vi "Photonics Measurements Launcher.vi"() -> ()   [LabVIEW 2019]
uses:
  Subsystems/Measurement/Typedefs/Measurement.Type--Enum.ctl
  Subsystems/Measurement/Typedefs/Configuration.SMU--Cluster.ctl
  Subsystems/SMU/Typedefs/Configuration--Cluster.ctl
  Subsystems/Measurement/Typedefs/Configuration.LIA--Cluster.ctl
  Subsystems/LIA/Typedefs/Configuration--Cluster.ctl
  Subsystems/Measurement/Typedefs/Configuration.OPM--Cluster.ctl
  Subsystems/OPM/Typedefs/Configuration--Cluster.ctl
  Subsystems/Measurement/Typedefs/Configuration.OPA--Cluster.ctl
  Subsystems/OPA/Typedefs/Configuration--Cluster.ctl
  Subsystems/Measurement/Typedefs/Configuration.XYStage--Cluster.ctl
  Subsystems/XYStage/Typedefs/Configuration--Cluster.ctl
  Subsystems/Measurement/Typedefs/Configuration.MC--Cluster.ctl
  Subsystems/MC/Typedefs/Configuration--Cluster.ctl
  Subsystems/Measurement.IVCurve/Typedefs/Configuration.Measurement--Cluster.ctl
  Subsystems/Measurement.WavelengthSweeping/Typedefs/Configuration.Measurement--Cluster.ctl
  Subsystems/Measurement.PhotocurrentMapping/Typedefs/Configuration.Measurement--Cluster.ctl
  Subsystems/Measurement.PhotocurrentMapping/Typedefs/Configuration.Axis--Cluster.ctl
  Subsystems/Measurement.Free/Measurement.Free.lvclass
  E:/UPWORK/Laser Tool/Laser/project/Subsystems/Measurement/Measurement.lvclass
  Subsystems/Measurement.Free.UI/Measurement.Free.UI.lvclass
  E:/UPWORK/Laser Tool/Laser/project/Subsystems/Measurement.UI/Measurement.UI.lvclass
  Subsystems/Measurement.IVCurve/Measurement.IVCurve.lvclass
  Subsystems/Measurement.IVCurve.UI/Measurement.IVCurve.UI.lvclass
  Subsystems/Measurement.WavelengthSweeping/Measurement.WavelengthSweeping.lvclass
  Subsystems/Measurement.WavelengthSweeping.UI/Measurement.WavelengthSweeping.UI.lvclass
  Subsystems/Measurement.PhotocurrentMapping/Measurement.PhotocurrentMapping.lvclass
  Subsystems/Measurement.PhotocurrentMapping.UI/Measurement.PhotocurrentMapping.UI.lvclass
  Subsystems/Measurement.Free/Typedefs/Configuration--Cluster.ctl
  Subsystems/Measurement.Free/Typedefs/Configuration.Hardware--Cluster.ctl
  Subsystems/Measurement.IVCurve/Typedefs/Configuration--Cluster.ctl
  Subsystems/Measurement.IVCurve/Typedefs/Configuration.Hardware--Cluster.ctl
  Subsystems/Measurement.WavelengthSweeping/Typedefs/Configuration--Cluster.ctl
  Subsystems/Measurement.WavelengthSweeping/Typedefs/Configuration.Hardware--Cluster.ctl
  Subsystems/Measurement.PhotocurrentMapping/Typedefs/Configuration--Cluster.ctl
  Subsystems/Measurement.PhotocurrentMapping/Typedefs/Configuration.Hardware--Cluster.ctl
  Subsystems/Measurement/Measurement.lvclass
  Subsystems/OPA.OrpheusHP/OPA.OrpheusHP.lvclass
  Subsystems/OPM.ThorlabsPM400/OPM.ThorlabsPM400.lvclass
  Subsystems/SMU/SMU.lvclass
  Subsystems/OPA/OPA.lvclass
  Subsystems/OPM/OPM.lvclass
  Subsystems/LIA/LIA.lvclass
  Subsystems/XYStage.KIM101/XYStage.KIM101.lvclass
  Subsystems/XYStage/XYStage.lvclass
  Subsystems/MC/MC.lvclass
panel:
  in  "OK":bool
  out "Measurements Tree":string(tree) caption="Chart A"
  in  "Add":bool
  in  "Remove":bool
  in  "Stop":bool
  in  "Start":bool
  in  "Measurement Parameters":T1(tab)
  in  "SMU step voltage, V":dbl=0.01 min=0.0 step=0.01 format="%.4f"
  in  "SMU stop voltage, V":dbl=2.0 min=0.0 step=0.01 format="%.4f"
  in  "SMU start voltage, V":dbl=1.0 min=0.0 step=0.01 format="%.4f"
  in  "I/V Curve Accumulation":u16=5 caption="Accumulation" step=1
  in  "Delay time, ms":u16=500 step=100
  in  "Monochromator\nwavelength offset, nm":dbl=50.0 step=20.0 format="%#_6f"
  in  "Delay time, ms":u16=500 step=100
  in  "W-Sweep Accumulation":u16=5 caption="Accumulation" step=1
  in  "Integration time, s":dbl=5.0 step=0.1
  in  "OPA number of points":u16 step=1
  in  "Scan resolution, nm":dbl=20.0 step=10.0 format="%#_6f"
  in  "Stop wavelength, nm":dbl=1000.0 step=20.0 format="%#_6f"
  in  "Start wavelength, nm":dbl=600.0 step=20.0 format="%#_6f"
  in  "SMU voltage, V":dbl=1.0 step=0.01 format="%#_6f"
  in  "P-Map Accumulation":u16=5 caption="Accumulation" step=1
  in  "Real world units":string="um"
  in  "Counts per unit":u32=1 step=100
  in  "Y Axis Step, units":dbl=250.0 step=100.0 format="%#_6f"
  in  "Y Axis Stop, units":dbl=10000.0 step=100.0 format="%#_6f"
  in  "Y Axis Start, units":dbl=-10000.0 step=100.0 format="%#_6f"
  in  "X Axis Step, units":dbl=250.0 step=100.0 format="%#_6f"
  in  "X Axis Stop, units":dbl=10000.0 step=100.0 format="%#_6f"
  in  "X Axis Start, units":dbl=-10000.0 step=100.0 format="%#_6f"
  in  "Sync":bool
  in  "Save":bool
  in  "Hardware Parameters":enum32{"Free"}(tab)
  in  "XYStage Enable":bool caption="XYStage"
  in  "Y Axis":string(combo)="Channel 2"
  in  "X Axis":string(combo)="Channel 1"
  in  "XYStage Refresh List":bool
  in  "XYStage Serial Number":string(combo) caption="Serial Number"
  in  "MC Enable":bool caption="MC"
  in  "MC Resource Name":refnum<visa-resource-name>="COM3" caption="Resource Name"
  in  "OPA Enable":bool caption="OPA"
  in  "OPA Refresh List":bool
  in  "OPA Serial Number":string(combo) caption="Serial Number"
  in  "OPM Enable":bool caption="OPM"
  in  "OPM Refresh List":bool
  in  "OPM Simulated":bool
  in  "OPM Resource Name":string(combo) caption="Resource Name"
  in  "LIA Enable":bool caption="LIA"
  in  "LIA Simulated":bool
  in  "LIA Resource Name":refnum<visa-resource-name>="GPIB0::8::INSTR" caption="Resource Name"
  in  "SMU Enable":bool caption="SMU"
  in  "SMU Channel":string(combo)="A" caption="Channel"
  in  "SMU Simulated":bool
  in  "SMU Resource Name":refnum<visa-resource-name>="GPIB0::26::INSTR" caption="Resource Name"
  in  "Close":bool
  out "Status":string
  out "Progress":u8(slide) scale=0.0..100.0
  # "XY Stage Controller"
  # "Monochromator"
  # "Optical Parametric Amplifier"
  # "Optical Power Monitor"
  # "Lock-In Amplifier"
  # "SMU"
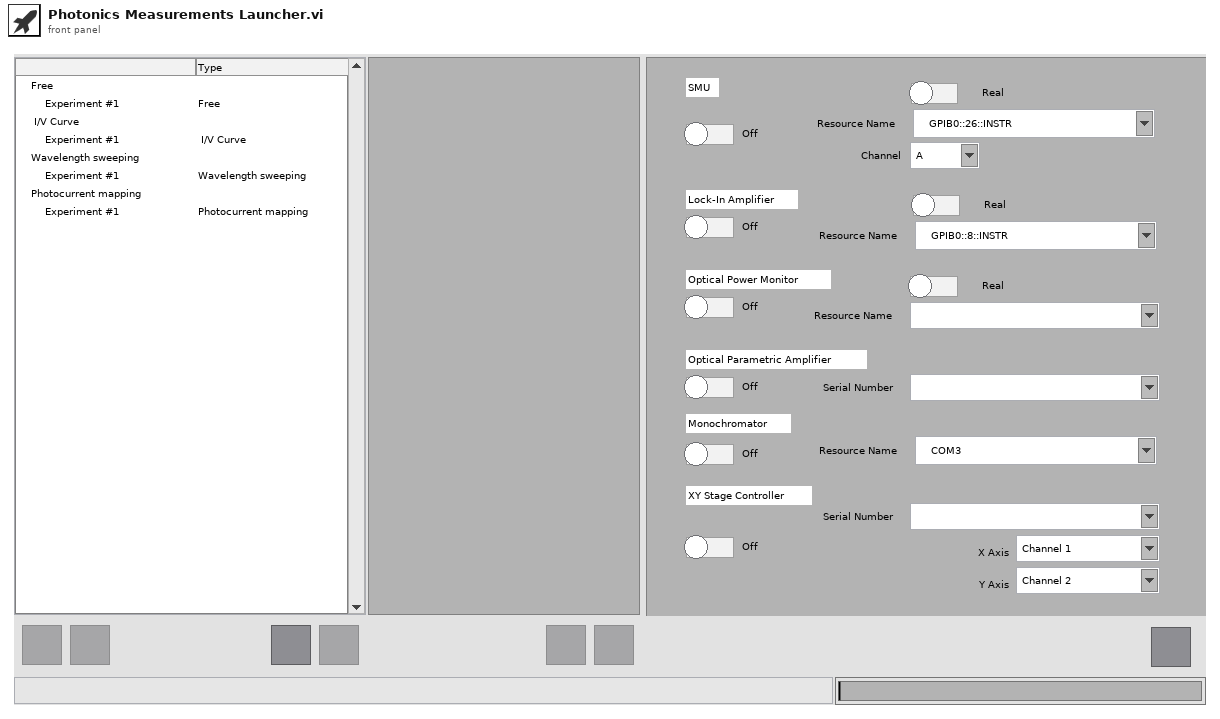
[diagram p1: front panel]
types:
  T1 = enum32{"Free", "I-V Curve", "Wavelength Sweeping", "Photocurrent mapping"}
  T2 = enum8{"Enabled", "Disabled", "Disabled and Grayed Out"}
  T3 = enum32{"Invalid", "Standard", "Closed", "Hidden", "Minimized", "Maximized"}
  T4 = enum32{"invalid app kind", "Development System", "Run Time System", "Student Edition", "Embedded LabVIEW", "Evaluation", "Custom"}
  T5 = typedef "Measurement.lvclass/Measurement.Type--Enum.ctl" = enum16{"Free", "I/V Curve", "Wavelength sweeping", "Photocurrent mapping"}
  T6 = typedef "LVPoint32TypeDef.ctl" = cluster{"Horizontal":i32, "Vertical":i32}
  T7 = typedef "Measurement.lvclass/Configuration.SMU--Cluster.ctl" = cluster{"Enable":bool, "SMU Model":string, "Configuration":T8}
  T8 = typedef "SMU.lvclass/Configuration--Cluster.ctl" = cluster{"VISA Resource":string, "Channel":string}
  T9 = typedef "Measurement.lvclass/Configuration.LIA--Cluster.ctl" = cluster{"Enable":bool, "LIA Model":string, "Configuration":T10}
  T10 = typedef "LIA.lvclass/Configuration--Cluster.ctl" = cluster{"VISA Resource":string}
  T11 = typedef "Measurement.lvclass/Configuration.OPM--Cluster.ctl" = cluster{"Enable":bool, "OPM Model":string, "Configuration":T12}
  T12 = typedef "OPM.lvclass/Configuration--Cluster.ctl" = cluster{"VISA Resource":string}
  T13 = typedef "Measurement.lvclass/Configuration.OPA--Cluster.ctl" = cluster{"Enable":bool, "OPA Model":string, "Configuration":T14}
  T14 = typedef "OPA.lvclass/Configuration--Cluster.ctl" = cluster{"Serial Number":string}
  T15 = typedef "Measurement.lvclass/Configuration.XYStage--Cluster.ctl" = cluster{"Enable":bool, "XYStage Model":string, "Configuration":T16}
  T16 = typedef "XYStage.lvclass/Configuration--Cluster.ctl" = cluster{"Serial Number":string, "X Axis":string, "Y Axis":string, "Real-World Units":string, "Counts per Unit":u32}
  T17 = typedef "Measurement.lvclass/Configuration.MC--Cluster.ctl" = cluster{"Enable":bool, "MC Model":string, "Configuration":T18}
  T18 = typedef "MC.lvclass/Configuration--Cluster.ctl" = cluster{"VISA Resource":string}
  T19 = typedef "Measurement.IVCurve.lvclass/Configuration.Measurement--Cluster.ctl" = cluster{"SMU Voltage Start, V":dbl, "SMU Voltage Stop, V":dbl, "SMU Voltage Step, V":dbl, "Delay time, ms":u16, "Accumulation":u16}
  T20 = typedef "Measurement.WavelengthSweeping.lvclass/Configuration.Measurement--Cluster.ctl" = cluster{"SMU Voltage, V":dbl, "Start wavelength, nm":dbl, "Stop wavelength, nm":dbl, "Scan resolution, nm":dbl, "Number or points":u16, "Integration time, sec":dbl, "Delay time, ms":u16, "Accumulation":u16, "Wavelength offset, nm":dbl}
  T21 = typedef "Measurement.PhotocurrentMapping.lvclass/Configuration.Measurement--Cluster.ctl" = cluster{"X":T22, "Y":T22, "Accumulation":u16}
  T22 = typedef "Measurement.PhotocurrentMapping.lvclass/Configuration.Axis--Cluster.ctl" = cluster{"Start, units":dbl, "Stop, units":dbl, "Step, units":dbl}
  T23 = cluster{"Core":cluster{"Current VI Reference":refnum<vi>, "Close Panel on Exit?":bool}, "Measurements Tree":refnum<vi>, "Measurement.Type":T5, "Configuration (variant)":variant, "Configuration":cluster{"Hardware":cluster{"SMU":T7, "LIA":T9, "OPM":T11, "OPA":T13, "XYStage":T15, "MC":T17}, "Measurement":cluster{"I/V Curve":T19, "W-Sweep":T20, "P-Map":T21}}}
  T24 = cluster{"Hardware":cluster{"SMU":T7, "LIA":T9, "OPM":T11, "OPA":T13, "XYStage":T15, "MC":T17}, "Measurement":cluster{"I/V Curve":T19, "W-Sweep":T20, "P-Map":T21}}
  T25 = cluster{"Current VI Reference":refnum<vi>, "Close Panel on Exit?":bool}
  T26 = typedef "Measurement.Free.lvclass/Configuration--Cluster.ctl" = cluster{"Measurement.Type":T5, "Hardware":T27}
  T27 = typedef "Measurement.Free.lvclass/Configuration.Hardware--Cluster.ctl" = cluster{"SMU":T7, "LIA":T9, "OPM":T11, "OPA":T13, "MC":T17}
  T28 = typedef "Measurement.IVCurve.lvclass/Configuration--Cluster.ctl" = cluster{"Measurement.Type":T5, "Hardware":T29, "Measurement":T19}
  T29 = typedef "Measurement.IVCurve.lvclass/Configuration.Hardware--Cluster.ctl" = cluster{"SMU":T7}
  T30 = typedef "Measurement.WavelengthSweeping.lvclass/Configuration--Cluster.ctl" = cluster{"Measurement.Type":T5, "Hardware":T31, "Measurement":T20}
  T31 = typedef "Measurement.WavelengthSweeping.lvclass/Configuration.Hardware--Cluster.ctl" = cluster{"SMU":T7, "LIA":T9, "OPM":T11, "OPA":T13, "MC":T17}
  T32 = typedef "Measurement.PhotocurrentMapping.lvclass/Configuration--Cluster.ctl" = cluster{"Measurement.Type":T5, "Hardware":T33, "Measurement":T21}
  T33 = typedef "Measurement.PhotocurrentMapping.lvclass/Configuration.Hardware--Cluster.ctl" = cluster{"SMU":T7, "LIA":T9, "XYStage":T15}
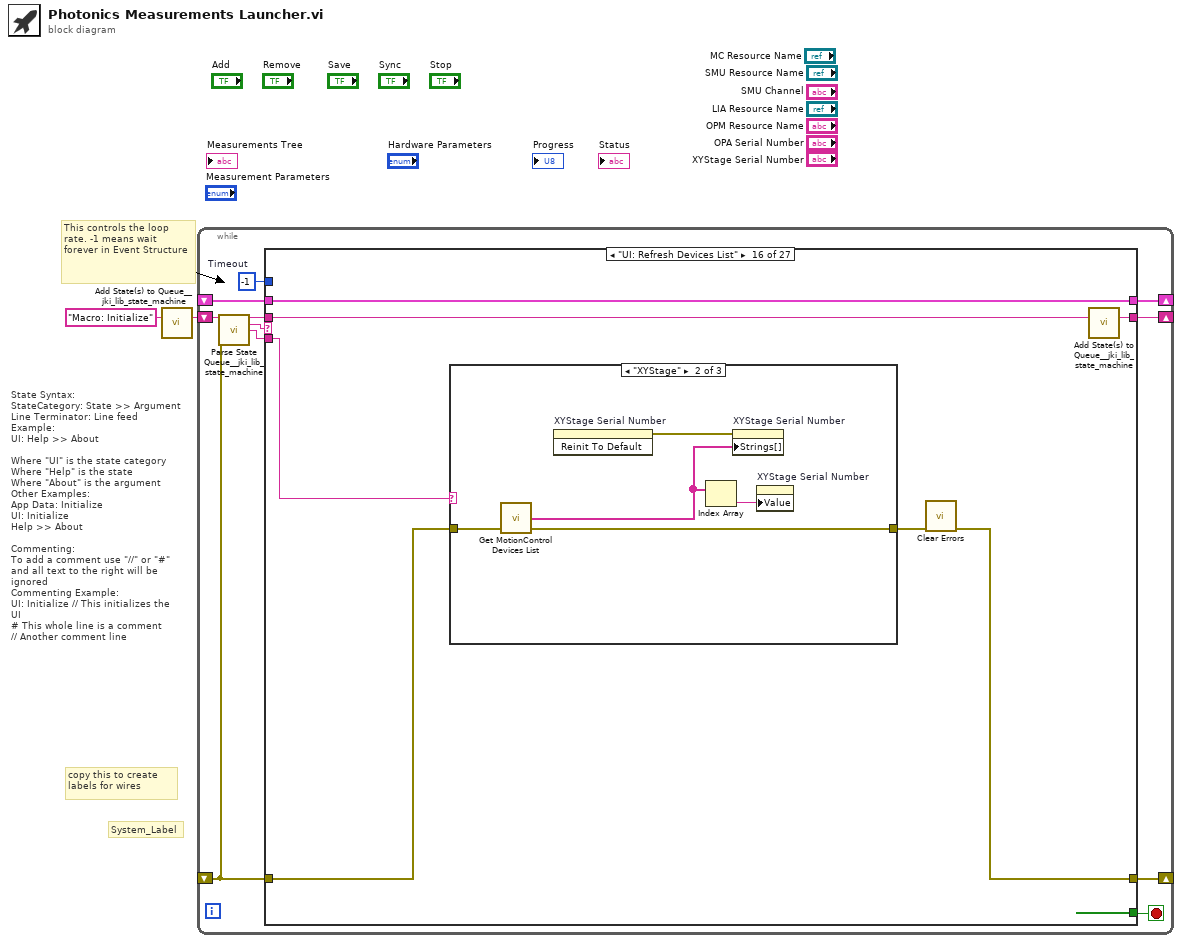
[diagram p0: block diagram]
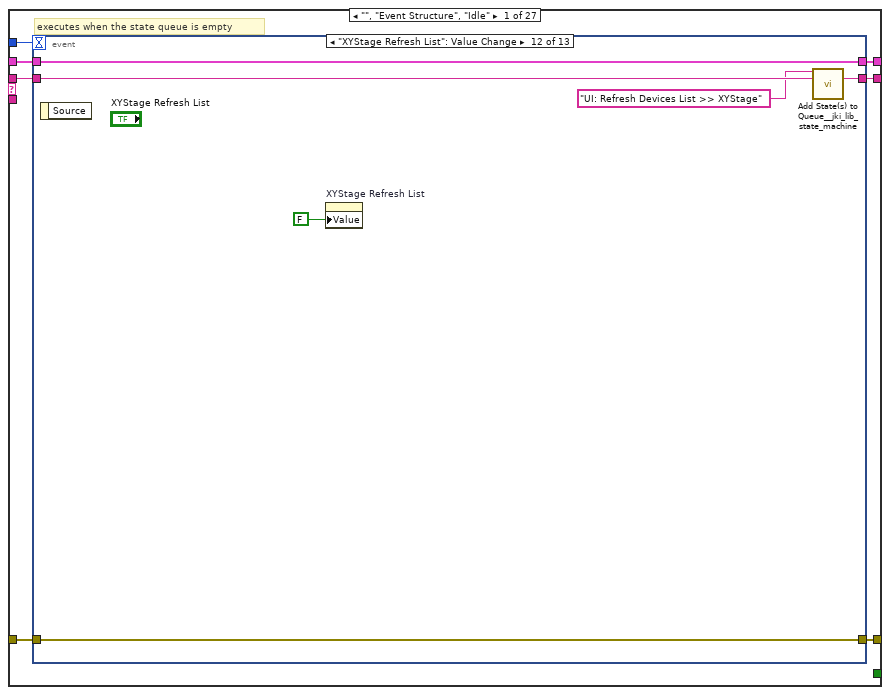
[diagram p2: hidden frame]
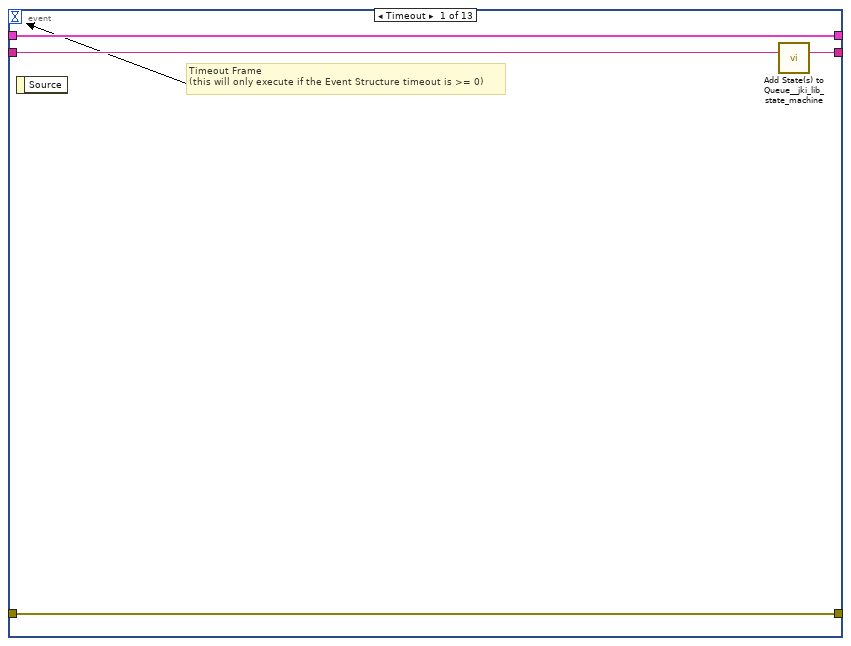
[diagram p3: hidden frame]
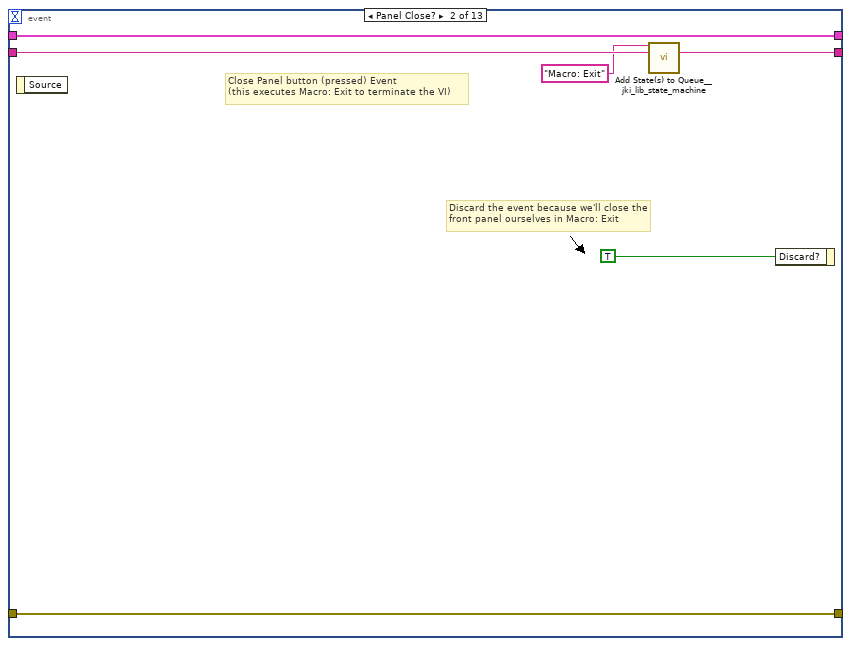
[diagram p4: hidden frame]
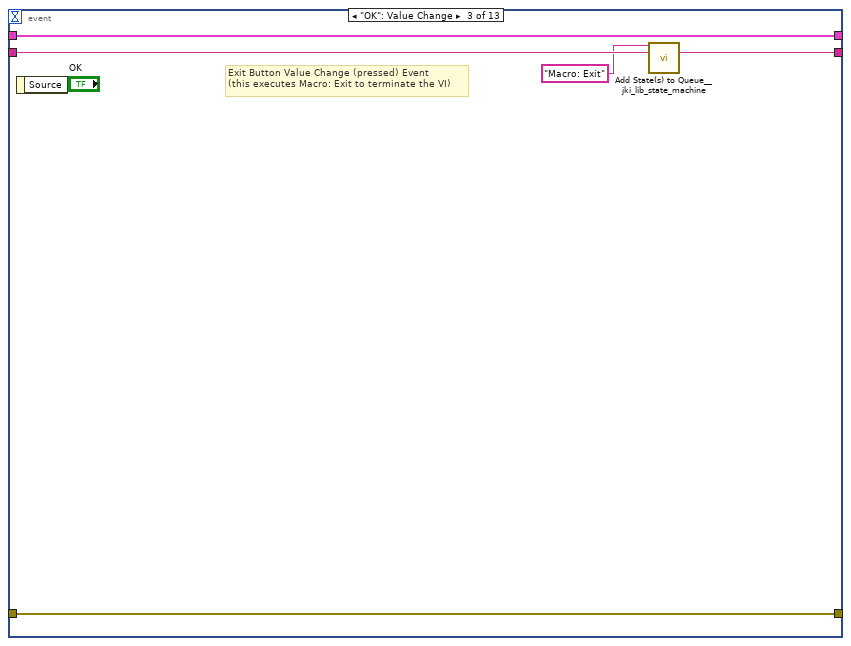
[diagram p5: hidden frame]
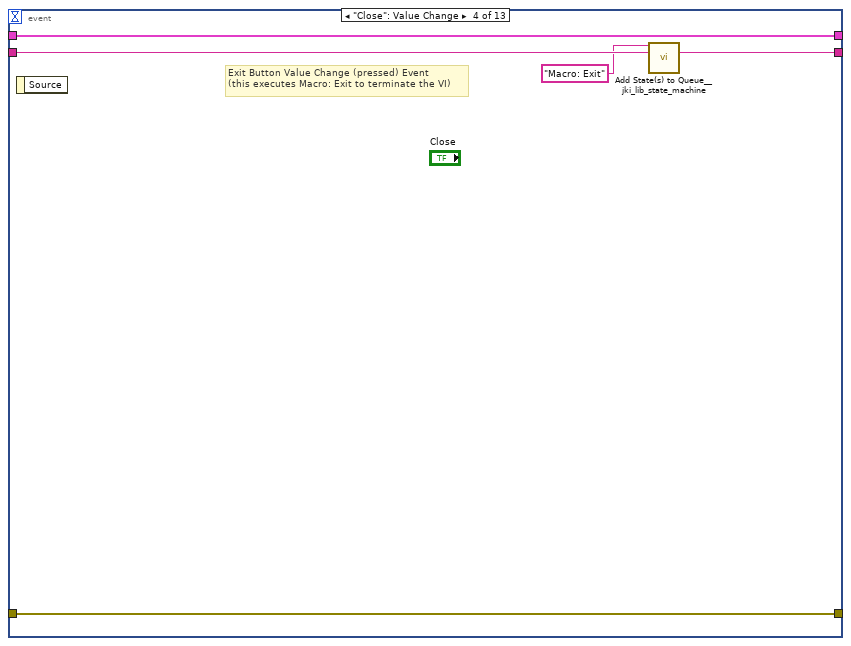
[diagram p6: hidden frame]
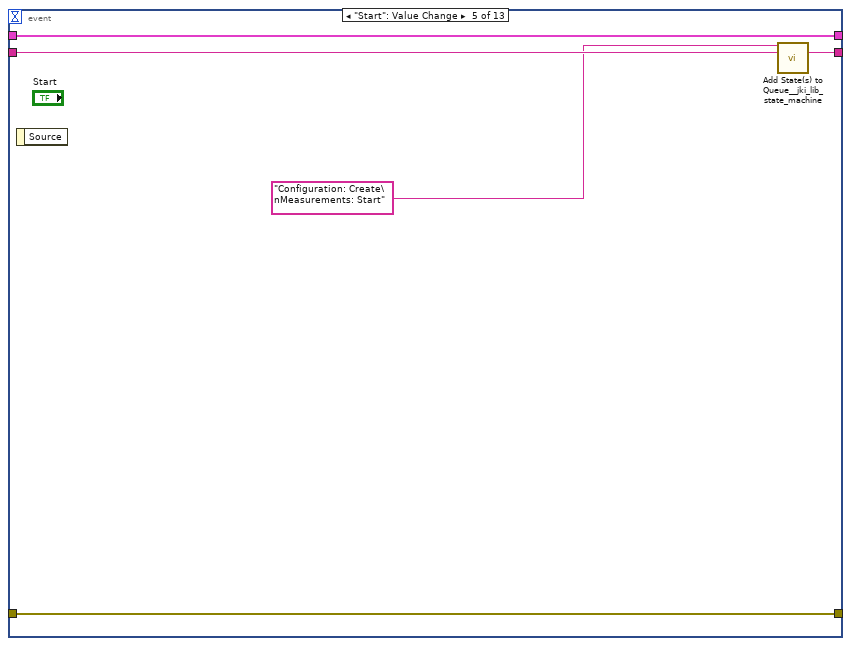
[diagram p7: hidden frame]
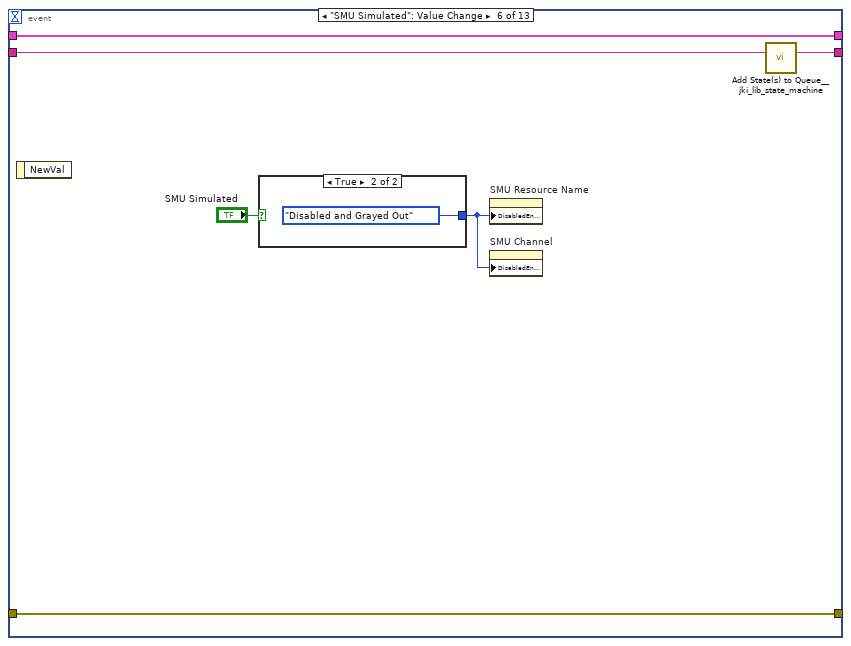
[diagram p8: hidden frame]
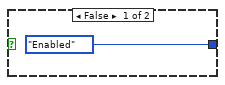
[diagram p9: hidden frame]
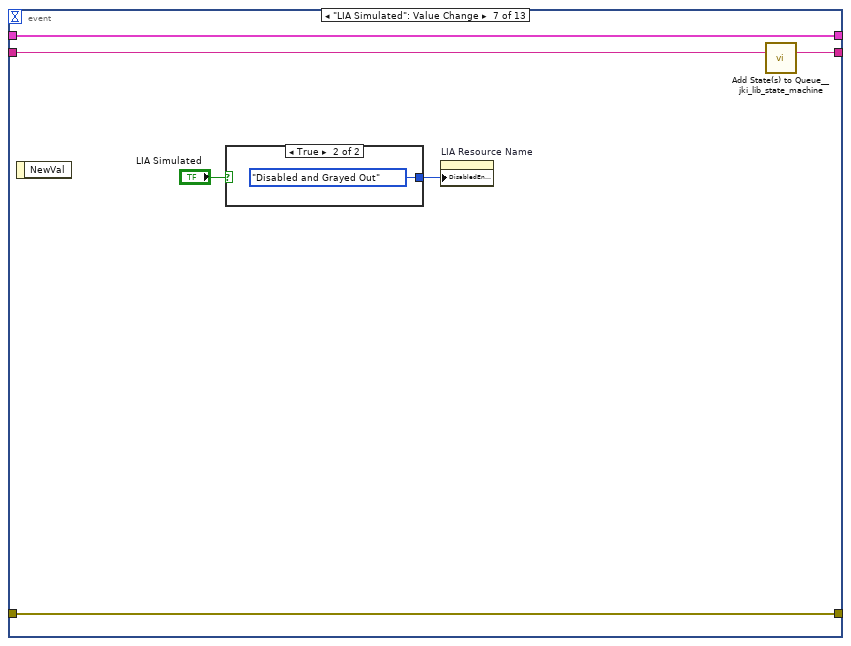
[diagram p10: hidden frame]
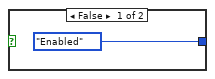
[diagram p11: hidden frame]
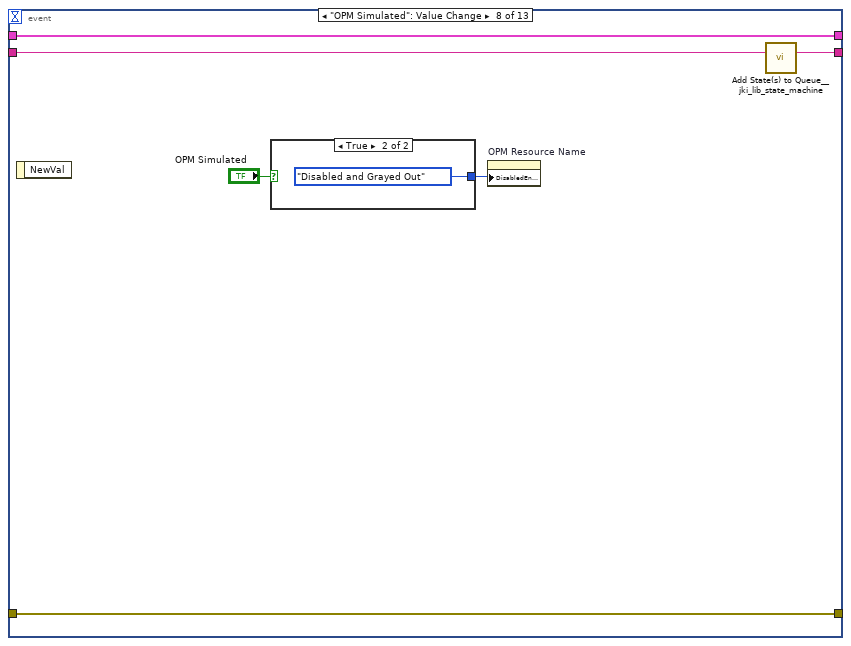
[diagram p12: hidden frame]
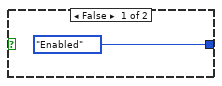
[diagram p13: hidden frame]
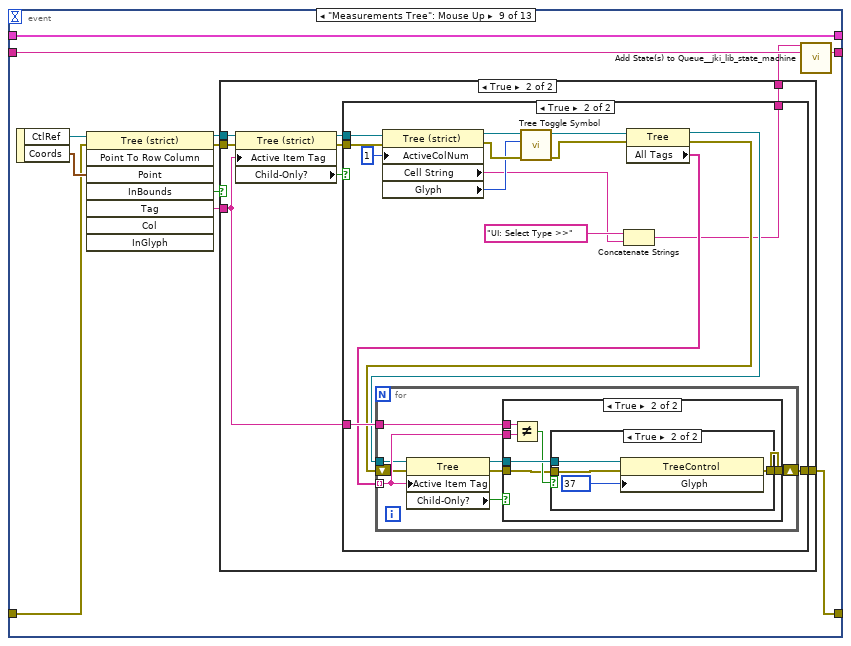
[diagram p14: hidden frame]
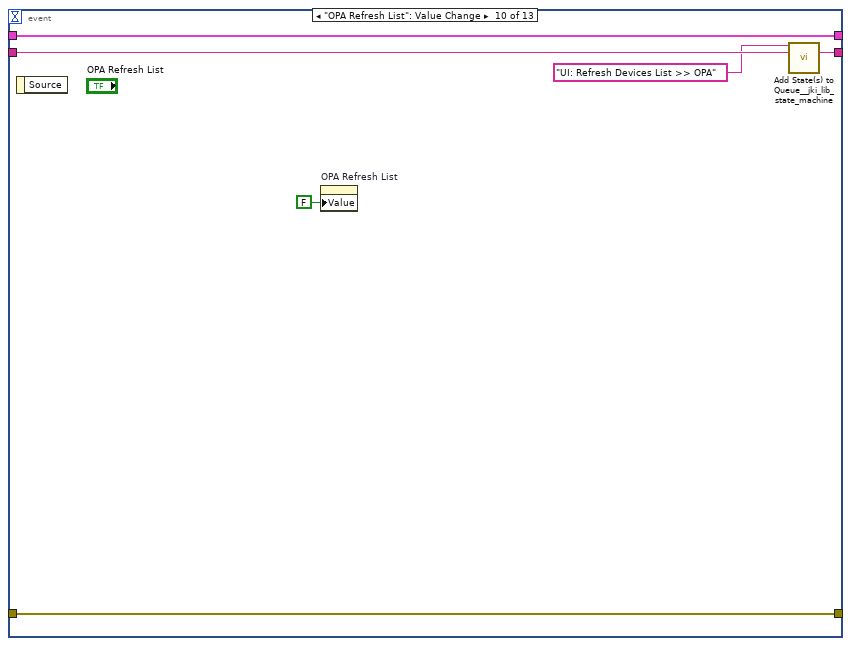
[diagram p19: hidden frame]
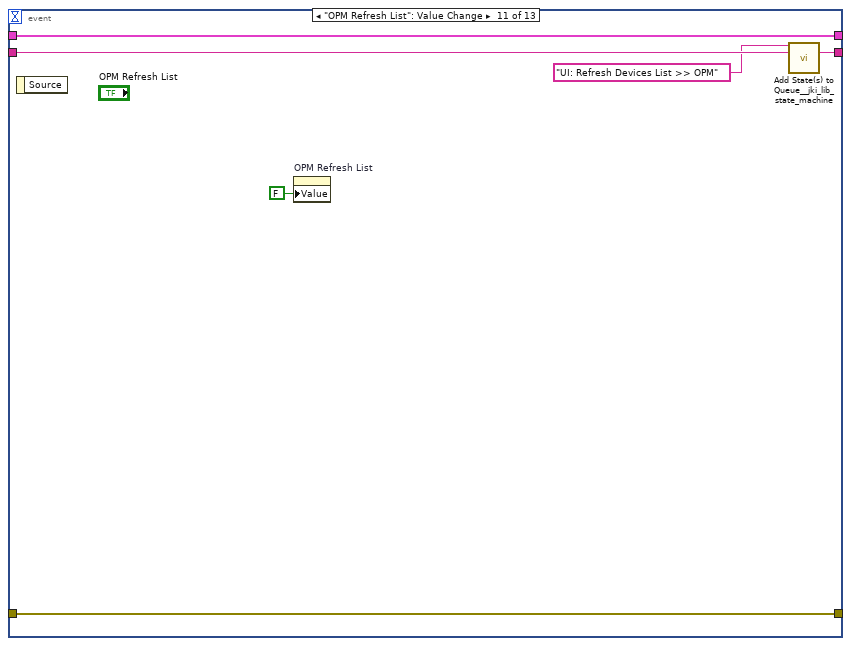
[diagram p20: hidden frame]
diagram:
  # "State Syntax:\nStateCategory: State >> Argument\nLine Terminator: Line feed\nExample:\nUI: Help >> About\n\nWhere \"UI\" is the state category\nWhere \"Help\" is the state\nWhere \"About\" is the argument\nOther Examples:\nApp Data: Initialize\nUI: Initialize\nHelp >> About\n\nCommenting:\nTo add a comment use \"//\" or \"#\" and all text to the right will be ignored\nCommenting Example:\nUI: Initialize // This initializes the UI\n# This whole line is a comment\n// Another comment line"
  # "copy this to create labels for wires"
  # "This controls the loop rate. -1 means wait forever in Event Structure"
  # "System_Label"
  n1 = call <vilib>:"Add State(s) to Queue__jki_lib_state_machine.vi"("State(s) in (\"\")"="Macro: Initialize") -> ("States Out"=w2:string)  [unwired: 14 in]
  n2 = while {
    shift-right: [w6] -> _
    shift-left: _ -> [w5]
    shift-right: [w9] -> _
    shift-left: _ -> [w3]
    shift-right: [w8] -> _
    shift-left: w2 -> [w10]
    stop <- w7 stop-if-true
    w4 = -1  # Timeout
    n3 = call <vilib>:"Parse State Queue__jki_lib_state_machine.vi"("State Queue"=w10, "Error In (no error)"=w3) -> ("Remaining States"=w12:string, "Current State"=w13:string, "Arguments"=w11:string)  [unwired: 11 in]
    n4 = case shown="\"UI: Refresh Devices List\"" w13 {
      selector: w13 -> [_ _ w158 _ _ _ _ _ _ _ _ _ _ _ _ _ _ _ _ _ _ _ _ _ _ _ _]
      tunnel: w12 -> [w20 w157 w162 w181 w187 w192 w196 w205 w211 w215 w220 w226 w231 w282 w305 w316 w338 w429 w481 w486 w496 w500 w509 w521 w527 w537 w637]
      tunnel: w11 -> [_ _ _ _ _ _ _ _ _ _ _ _ w227 _ w300 w313 w332 w432 _ _ _ _ _ _ _ w534 w634]
      tunnel: w5 -> [w18 w154 w160 w174 w184 w190 w193 _ w206 w212 w218 w223 w228 w279 w303 w314 w334 w431 w478 w483 w493 w497 w507 w518 w524 w533 w633]
      tunnel: [w17 w155 w164 w178 errorcluster {"status"=FALSE, "code"=0, "source"=""} ("error out") w189 w194 w202 w207 w213 w217 w224 w229 w263 w301 w310 w335 w428 w479 w484 w494 w498 w502 w519 w525 w535 w635] -> w9
      tunnel: w3 -> [w16 w155 w163 w178 w183 w189 w194 w202 w208 w213 w217 w224 w229 w268 w302 w312 w336 w428 w479 w484 w494 w498 w503 w519 w525 w535 w635]
      tunnel: [w19 w156 w161 w180 w186 w191 w195 w204 w210 w214 w219 w225 w230 w281 w304 w315 w337 w433 w480 w485 w495 w499 w508 w520 w526 w536 w636] -> w8
      tunnel: [_ _ _ _ _ TRUE _ _ _ _ _ _ _ _ _ _ _ _ _ _ _ _ _ _ _ _ _] -> w7
      tunnel: [w15 w154 w160 w179 w184 w190 w193 w203 w206 w212 w218 w223 w228 w279 w303 w314 w334 w430 w478 w483 w493 w497 w507 w518 w524 w532 w632] -> w6
      tunnel: w4 -> [w14 _ _ _ _ _ _ _ _ _ _ _ _ _ _ _ _ _ _ _ _ _ _ _ _ _ _]
      frame "", "Event Structure", "Idle" {
        # "executes when the state queue is empty"
        n5 = event shown="[11] \"XYStage Refresh List\": Value Change" {
          selector: _ -> [_ _ _ _ _ _ _ _ _ _ _ _ _]
          dyn-events: _ -> [_ _ _ _ _ _ _ _ _ _ _ _ _]
          timeout: w14 -> [_ _ _ _ _ _ _ _ _ _ _ _ _]
          tunnel: w20 -> [w24 w30 w35 w40 w43 w47 w57 w65 w79 w133 w139 w145 w150]
          tunnel: [w23 w29 w34 w39 w44 w48 w58 w66 w80 w132 w138 w144 w151] -> w19
          tunnel: w18 -> [w21 w27 w32 w37 w45 w49 w59 w67 w81 w130 w136 w142 w152]
          tunnel: [w22 w28 w33 w38 w42 w46 w56 w64 w72 w131 w137 w143 w153] -> w17
          tunnel: w16 -> [w22 w28 w33 w38 w42 w46 w56 w64 w71 w131 w137 w143 w153]
          tunnel: [w21 w27 w32 w37 w45 w49 w59 w67 w81 w130 w136 w142 w152] -> w15
          event Timeout {
            # "Timeout Frame\n(this will only execute if the Event Structure timeout is >= 0)"
            n6 = event-data() -> ()  [unwired: 1 in, 1 out]
            n7 = call <vilib>:"Add State(s) to Queue__jki_lib_state_machine.vi"("State(s) in (\"\")"=w24) -> ("States Out"=w23:string)  [unwired: 14 in]
          }
          event Panel Close? {
            # "Discard the event because we'll close the front panel ourselves in Macro: Exit"
            # "Close Panel button (pressed) Event\n(this executes Macro: Exit to terminate the VI)"
            n8 = event-data() -> ()  [unwired: 1 in, 1 out]
            n9 = call <vilib>:"Add State(s) to Queue__jki_lib_state_machine.vi"("State(s) in Front (\"\")"="Macro: Exit", "State(s) in (\"\")"=w30) -> ("States Out"=w29:string)  [unwired: 13 in]
            n10 = event-data("Discard?"=TRUE) -> ()  [unwired: 1 in, 1 out]
          }
          event "OK": Value Change {
            # "Exit Button Value Change (pressed) Event\n(this executes Macro: Exit to terminate the VI)"
            n11 = event-data() -> ()  [unwired: 1 in, 1 out]
            n12 = call <vilib>:"Add State(s) to Queue__jki_lib_state_machine.vi"("State(s) in Front (\"\")"="Macro: Exit", "State(s) in (\"\")"=w35) -> ("States Out"=w34:string)  [unwired: 13 in]
          }
          event "Close": Value Change {
            # "Exit Button Value Change (pressed) Event\n(this executes Macro: Exit to terminate the VI)"
            n13 = event-data() -> ()  [unwired: 1 in, 1 out]
            n14 = call <vilib>:"Add State(s) to Queue__jki_lib_state_machine.vi"("State(s) in Front (\"\")"="Macro: Exit", "State(s) in (\"\")"=w40) -> ("States Out"=w39:string)  [unwired: 13 in]
          }
          event "Start": Value Change {
            n15 = event-data() -> ()  [unwired: 1 in, 1 out]
            n16 = call <vilib>:"Add State(s) to Queue__jki_lib_state_machine.vi"("State(s) in Front (\"\")"="Configuration: Create\nMeasurements: Start" ("State(s) in Front (\"\")"), "State(s) in (\"\")"=w43) -> ("States Out"=w44:string)  [unwired: 13 in]
          }
          event "SMU Simulated": Value Change {
            n17 = event-data() -> ()  [unwired: 1 in, 1 out]
            n18 = case shown="True" "SMU Simulated" {
              tunnel: [T2."Enabled" ("Disabled") T2."Disabled and Grayed Out" ("Disabled")] -> w51
              frame False {
              }
              frame True {
              }
            }
            n19 = property on="SMU Resource Name" class="VISAName"("DisabledEnum"=w51) -> ()  [unwired: 2 in, 2 out]
            n20 = property on="SMU Channel" class="CmbBox"("DisabledEnum"=w51) -> ()  [unwired: 2 in, 2 out]
            n21 = call <vilib>:"Add State(s) to Queue__jki_lib_state_machine.vi"("State(s) in (\"\")"=w47) -> ("States Out"=w48:string)  [unwired: 14 in]
          }
          event "LIA Simulated": Value Change {
            n22 = event-data() -> ()  [unwired: 1 in, 1 out]
            n23 = case shown="True" "LIA Simulated" {
              tunnel: [T2."Enabled" ("Disabled") T2."Disabled and Grayed Out" ("Disabled")] -> w55
              frame False {
              }
              frame True {
              }
            }
            n24 = property on="LIA Resource Name" class="VISAName"("DisabledEnum"=w55) -> ()  [unwired: 2 in, 2 out]
            n25 = call <vilib>:"Add State(s) to Queue__jki_lib_state_machine.vi"("State(s) in (\"\")"=w57) -> ("States Out"=w58:string)  [unwired: 14 in]
          }
          event "OPM Simulated": Value Change {
            n26 = event-data() -> ()  [unwired: 1 in, 1 out]
            n27 = case shown="True" "OPM Simulated" {
              tunnel: [T2."Enabled" ("Disabled") T2."Disabled and Grayed Out" ("Disabled")] -> w63
              frame False {
              }
              frame True {
              }
            }
            n28 = property on="OPM Resource Name" class="CmbBox"("DisabledEnum"=w63) -> ()  [unwired: 2 in, 2 out]
            n29 = call <vilib>:"Add State(s) to Queue__jki_lib_state_machine.vi"("State(s) in (\"\")"=w65) -> ("States Out"=w66:string)  [unwired: 14 in]
          }
          event "Measurements Tree": Mouse Up {
            n30 = event-data() -> ("CtlRef"=w78:refnum<vi>, "Coords"=w77:T6)  [unwired: 1 in]
            n31 = invoke class="Tree (strict)" method="Point To Row Column"(reference=w78, error in=w71, "Point"=w77) -> (reference out=w75:refnum<vi>, error out=w74:errorcluster, "InBounds"=w76:bool, "Tag"=w73:string)  [unwired: 5 in, 4 out]
            n32 = case shown="True" w76 {
              tunnel: w75 -> [_ w90]
              tunnel: w74 -> [w82 w89]
              tunnel: w73 -> [_ w85]
              tunnel: [w82 w84] -> w72
              tunnel: [_ w83] -> w70
              frame False {
              }
              frame True {
                n33 = property class="Tree (strict)"(reference=w90, error in=w89, "Active Item Tag"=w85) -> (reference out=w87:refnum<vi>, error out=w86:errorcluster, "Child-Only?"=w88:bool)
                n34 = case shown="True" w88 {
                  tunnel: w87 -> [_ w106]
                  tunnel: w86 -> [w91 w107]
                  tunnel: w85 -> [_ w99]
                  tunnel: [w91 w93] -> w84
                  tunnel: [_ w92] -> w83
                  frame False {
                  }
                  frame True {
                    n35 = property class="Tree (strict)"(reference=w106, error in=w107, "ActiveColNum"=1 ("Active Cell:Active Column Number")) -> (reference out=w104:refnum<vi>, error out=w103:errorcluster, "Cell String"=w100:string, "Glyph"=w102:i32)
                    n36 = call "Tree Toggle Symbol.vi"("error in (no error)"=w103, "Symbol in"=w102, "TreeControl in"=w104) -> ("error out"=w97:errorcluster, "TreeControl out"=w98:refnum<vi>)  [unwired: 5 in, 2 out]
                    n37 = Concatenate Strings("UI: Select Type >>", w100) -> (w92:string)
                    n38 = property class="Tree"(reference=w98, error in=w97) -> (reference out=w96:refnum<vi>, error out=w95:errorcluster, "All Tags"=w94:string[])
                    n39 = for {
                      tunnel: w94 -> [w113] mode=indexing
                      tunnel: w99 -> [w114]
                      tunnel: w96 -> [w111]
                      shift-right: [w108] -> w93
                      shift-left: w95 -> [w110]
                      n40 = property class="Tree"(reference=w111, error in=w110, "Active Item Tag"=w113) -> (reference out=w112:refnum<vi>, error out=w109:errorcluster, "Child-Only?"=w115:bool)
                      n41 = case shown="True" w115 {
                        tunnel: w114 -> [_ w122]
                        tunnel: w113 -> [_ w121]
                        tunnel: w112 -> [_ w120]
                        tunnel: w109 -> [w116 w118]
                        tunnel: [w116 w117] -> w108
                        frame False {
                        }
                        frame True {
                          n42 = Not Equal?(x=w122, y=w121) -> (x != y?=w119:bool)
                          n43 = case shown="True" w119 {
                            tunnel: w120 -> [_ w127]
                            tunnel: w118 -> [w123 w125]
                            tunnel: [w123 w124] -> w117
                            frame False {
                            }
                            frame True {
                              n44 = property class="TreeControl"(reference=w127, error in=w125, "Glyph"=37) -> (error out=w124:errorcluster)  [unwired: 1 out]
                            }
                          }
                        }
                      }
                    }
                  }
                }
              }
            }
            n45 = call <vilib>:"Add State(s) to Queue__jki_lib_state_machine.vi"("State(s) in Front (\"\")"=w70, "State(s) in (\"\")"=w79) -> ("States Out"=w80:string)  [unwired: 13 in]
          }
          event "OPA Refresh List": Value Change {
            n46 = event-data() -> ()  [unwired: 1 in, 1 out]
            n47 = property on="OPA Refresh List" class="Bool (strict)"("Value"=FALSE ("OPA Refresh List")) -> ()  [unwired: 2 in, 2 out]
            n48 = call <vilib>:"Add State(s) to Queue__jki_lib_state_machine.vi"("State(s) in Front (\"\")"="UI: Refresh Devices List >> OPA", "State(s) in (\"\")"=w133) -> ("States Out"=w132:string)  [unwired: 13 in]
          }
          event "OPM Refresh List": Value Change {
            n49 = event-data() -> ()  [unwired: 1 in, 1 out]
            n50 = property on="OPM Refresh List" class="Bool (strict)"("Value"=FALSE ("OPM Refresh List")) -> ()  [unwired: 2 in, 2 out]
            n51 = call <vilib>:"Add State(s) to Queue__jki_lib_state_machine.vi"("State(s) in Front (\"\")"="UI: Refresh Devices List >> OPM", "State(s) in (\"\")"=w139) -> ("States Out"=w138:string)  [unwired: 13 in]
          }
          event "XYStage Refresh List": Value Change {
            n52 = event-data() -> ()  [unwired: 1 in, 1 out]
            n53 = property on="XYStage Refresh List" class="Bool (strict)"("Value"=FALSE ("OPM Refresh List")) -> ()  [unwired: 2 in, 2 out]
            n54 = call <vilib>:"Add State(s) to Queue__jki_lib_state_machine.vi"("State(s) in Front (\"\")"="UI: Refresh Devices List >> XYStage", "State(s) in (\"\")"=w145) -> ("States Out"=w144:string)  [unwired: 13 in]
          }
          event "SMU Enable", "LIA Enable", "OPM Enable", "OPA Enable", "MC Enable", "XYStage Enable": Value Change {
            n55 = event-data() -> ("CtlRef"=w146:refnum<vi>)  [unwired: 1 in]
            n56 = property class="Bool (strict)"(reference=w146) -> ("Caption.Text"=w148:string)  [unwired: 1 in, 2 out]
            n57 = Concatenate Strings("UI: Enable/Disable >> ", w148) -> (w147:string)
            n58 = call <vilib>:"Add State(s) to Queue__jki_lib_state_machine.vi"("State(s) in Front (\"\")"=w147, "State(s) in (\"\")"=w150) -> ("States Out"=w151:string)  [unwired: 13 in]
          }
        }
      }
      frame "---------- Core ----------" {
        # "Do not put any code in this frame.\n(it is a separator no-op)"
        n59 = call <vilib>:"Add State(s) to Queue__jki_lib_state_machine.vi"("State(s) in (\"\")"=w157) -> ("States Out"=w156:string)  [unwired: 14 in]
      }
      frame Default {
        w167 = 42 items=["No error", "Argument error", "Memory is full", "Out of zone", "End of file", "File already open", "Generic file I/O error", "File not found", "File permission error", "Disk is full", "Duplicate path", "Too many files open", "System feature not enabled", "Resource file not found", "Cannot add resource", "Resource not found", "Image not found", "Image memory error", "Pen does not exist", "Config type invalid", "Config token not found", "Config parse error", "Config memory error", "Bad external code format", "Bad external code offset", "External code not present", "Null window", "Destroy window error", "Null menu", "Print aborted", "Bad print record", "Print driver error", "Windows error during printing", "Memory error during printing", "Print dialog error", "Generic print error", "Invalid device refnum", "Device not found", "Device parameter error", "Device unit error", "Cannot open device", "Device call aborted", "Generic error", "Cancelled by user", "Object ID too low", "Object ID too high", "Object not in heap", "Unknown heap", "Unknown object (invalid DefProc)", "Unknown object (DefProc not in table)", "Message out of range", "Invalid (null) method", "Unknown message", "Manager call not supported", "Bad address", "Network operation in progress", "Network operation timed out", "Connection is busy", "Network attribute not supported", "Network error", "Address in use", "System out of memory", "Connection aborted", "Connection refused", "Not connected", "Already connected", "Connection closed", "Initialization error (interapplication manager)", "Bad occurrence", "Wait on unbound occurrence handler", "Occurrence queue overflow", "Datalog type conflict", "Unused", "Unrecognized type (interapplication manager)", "Memory corrupt", "Failed to make temporary DLL", "Old CIN version", "Drag socket not found", "Failed to load drop-object", "Failed to register OLE object", "Failed to release OLE object", "Format specifier type mismatch", "Unknown format specifier", "Too few format specifiers", "Too many format specifiers", "Scan failed", "Newer CIN version", "Error converting to variant", "Runtime menu error", "Password tampered", "Variant attribute not found", "Incompatible variant data type", "Event data is not available", "Event Store is not present", "Occurrence is not found", "Event Queue is not created", "Event info is not available", "Refnum passed is NULL", "Error retrieving Class GUID", "Error retrieving CoClass GUID", "Error retrieving TypeLib GUID.", "Bad built application magic bytes.", "Specific driver is different from the specific driver associated with the Logical Name.", "There is no session opened to the class driver.", "Max Error", "MAX - Error with config objects", "MAX - Error loading configuration", "MAX - Group not supported"]
        # "Current State"
        # "Do not delete, rename, or modify this frame.\n(this is used to capture unhandled states and typos)"
        # "Handle mistyped state name (developer tool)"
        n60 = Format Into String(format string="Software Exception: Unhandled State \"%s\"." ("message"), error in=w163, w158) -> (resulting string=w166:string, error out=w165:errorcluster)  [unwired: 1 in]
        n61 = call <vilib>:"Error Cluster From Error Code.vi"("show call chain? (False)"=TRUE, "error in (no error)"=w165, "error message (\"\")"=w166, "error code (0)"=w167) -> ("error out"=w164:errorcluster)  [unwired: 5 in]
        n62 = call <vilib>:"Add State(s) to Queue__jki_lib_state_machine.vi"("State(s) in (\"\")"=w162) -> ("States Out"=w161:string)  [unwired: 14 in]
      }
      frame "Initialize Core Data" {
        # "Do not delete, rename, or modify this frame.\n(this is used to determine panel behavior on exit)"
        # "originally closed?"
        # "exe?"
        # "If panel starts closed or is an EXE, then close it when we exit"
        n63 = property class="VI"() -> ("FP.State"=w171:T3)  [unwired: 2 in, 2 out]
        n64 = property class="App"() -> ("App.Kind"=w177:T4)  [unwired: 2 in, 2 out]
        n65 = control-ref of="Current VI Reference"() -> (w172:refnum<vi>)
        n66 = Equal?(x=w171, y=T3."Closed" ("Front Panel Window:State")) -> (x = y?=w169:bool)
        n67 = Equal?(x=w177, y=T4."Run Time System" ("Application:Kind")) -> (x = y?=w175:bool)
        n68 = Or(x=w169, y=w175) -> (x .or. y?=w173:bool)
        n69 = Bundle By Name(cluster=w174, "Core.Current VI Reference"=w172, "Core.Close Panel on Exit?"=w173) -> (w179:T23)
        n70 = call <vilib>:"Add State(s) to Queue__jki_lib_state_machine.vi"("State(s) in (\"\")"=w181) -> ("States Out"=w180:string)  [unwired: 14 in]
      }
      frame "Error Handler" {
        # "Unhandled Error -- Display it"
        # "Handle any errors here.\nYou can also output any states to clean-up after errors occur"
        # "Clear error"
        n71 = call <vilib>:"General Error Handler.vi"("error in (no error)"=w183) -> ()  [unwired: 10 in, 5 out]
        n72 = call <vilib>:"Add State(s) to Queue__jki_lib_state_machine.vi"("State(s) in Front (\"\")"="/* Post Error States", "State(s) in (\"\")"=w187) -> ("States Out"=w186:string)  [unwired: 13 in]
      }
      frame "Exit" {
        # "Do not put any code in this frame.\n(No errors that occur here will be handled.)"
        n73 = call <vilib>:"Add State(s) to Queue__jki_lib_state_machine.vi"("State(s) in (\"\")"=w192) -> ("States Out"=w191:string)  [unwired: 14 in]
      }
      frame "---------- Data ----------" {
        # "Do not put any code in this frame.\n(It is a separator no-op. You can make a copy of this frame to create a new Data frame)"
        n74 = call <vilib>:"Add State(s) to Queue__jki_lib_state_machine.vi"("State(s) in (\"\")"=w196) -> ("States Out"=w195:string)  [unwired: 14 in]
      }
      frame "Data: Initialize" {
        w197 = T24 {"Hardware"={"SMU"={"Enable"=FALSE, "SMU Model"="", "Configuration"={"VISA Resource"="", "Channel"=""}}, "LIA"={"Enable"=FALSE, "LIA Model"="", "Configuration"={"VISA Resource"=""}}, "OPM"={"Enable"=FALSE, "OPM Model"="", "Configuration"={"VISA Resource"=""}}, "OPA"={"Enable"=FALSE, "OPA Model"="", "Configuration"={"Serial Number"=""}}, "XYStage"={"Enable"=FALSE, "XYStage Model"="", "Configuration"={"Serial Number"="", "X Axis"="", "Y Axis"="", "Real-World Units"="", "Counts per Unit"=1}}, "MC"={"Enable"=FALSE, "MC Model"="", "Configuration"={"VISA Resource"=""}}}, "Measurement"={"I/V Curve"={"SMU Voltage Start, V"=0.0, "SMU Voltage Stop, V"=0.0, "SMU Voltage Step, V"=0.0, "Delay time, ms"=0, "Accumulation"=0}, "W-Sweep"={"SMU Voltage, V"=0.0, "Start wavelength, nm"=0.0, "Stop wavelength, nm"=0.0, "Scan resolution, nm"=0.0, "Number or points"=0, "Integration time, sec"=0.0, "Delay time, ms"=0, "Accumulation"=0, "Wavelength offset, nm"=0.0}, "P-Map"={"X"={"Start, units"=-10000.0, "Stop, units"=10000.0, "Step, units"=250.0}, "Y"={"Start, units"=-10000.0, "Stop, units"=10000.0, "Step, units"=250.0}, "Accumulation"=5}}}  # Configuration
        w198 = variant  # Configuration (variant)
        w199 = Measurement.Type--Enum."Free"  # Measurement.Type
        w201 = T25 {"Current VI Reference"=refnum, "Close Panel on Exit?"=FALSE}  # Core
        # "do not delete - used by framework"
        # "Data names and types of shift register data are defined by this bundle."
        # "Initialize the shift-register data, here.\n(data names are defined by what you wire into the bundle function)"
        n75 = control-ref of="Measurements Tree"() -> (w200:refnum<vi>)
        n76 = Bundle("Core"=w201, "Measurements Tree"=w200, "Measurement.Type"=w199, "Configuration (variant)"=w198, "Configuration"=w197) -> (w203:T23)  [unwired: 1 in]
        n77 = call <vilib>:"Add State(s) to Queue__jki_lib_state_machine.vi"("State(s) in (\"\")"=w205) -> ("States Out"=w204:string)  [unwired: 14 in]
      }
      frame "Data: Cleanup" {
        # "Cleanup any data and references, here.\n(this is called automatically, by the Macro: Exit)"
        n78 = Unbundle By Name(w206) -> ("Core.Current VI Reference"=w209:refnum<vi>)
        n79 = Close Reference(reference=w209, error in (no error)=w208) -> (error out=w207:errorcluster)
        n80 = call <vilib>:"Add State(s) to Queue__jki_lib_state_machine.vi"("State(s) in (\"\")"=w211) -> ("States Out"=w210:string)  [unwired: 14 in]
      }
      frame "---------- UI ----------" {
        # "Do not put any code in this frame.\n(It is a separator no-op. You can make a copy of this frame to create a new UI frame)"
        n81 = call <vilib>:"Add State(s) to Queue__jki_lib_state_machine.vi"("State(s) in (\"\")"=w215) -> ("States Out"=w214:string)  [unwired: 14 in]
      }
      frame "UI: Initialize" {
        # "Initialize the User Interface, here.\n(this is called automatically, by the Macro: Init)"
        n82 = call <vilib>:"Add State(s) to Queue__jki_lib_state_machine.vi"("State(s) in Front (\"\")"="UI: Tree Init\nUI: Initial State\nUI: Refresh Devices List >> OPM\nUI: Refresh Devices List >> OPA\nUI: Refresh Devices List >> XYStage\nUI: Select Type >> Free", "State(s) in (\"\")"=w220) -> ("States Out"=w219:string)  [unwired: 13 in]
      }
      frame "UI: Initial State" {
        w221 = FALSE ("SMU Simulated")
        w222 = TRUE ("SMU Enable")
        n83 = property on="SMU Enable" class="Bool (strict)"("Value"=w222) -> ()  [unwired: 2 in, 2 out]
        n84 = property on="LIA Enable" class="Bool (strict)"("Value"=w222) -> ()  [unwired: 2 in, 2 out]
        n85 = property on="OPM Enable" class="Bool (strict)"("Value"=w222) -> ()  [unwired: 2 in, 2 out]
        n86 = property on="OPA Enable" class="Bool (strict)"("Value"=w222) -> ()  [unwired: 2 in, 2 out]
        n87 = property on="MC Enable" class="Bool (strict)"("Value"=w222) -> ()  [unwired: 2 in, 2 out]
        n88 = property on="XYStage Enable" class="Bool (strict)"("Value"=w222) -> ()  [unwired: 2 in, 2 out]
        n89 = property on="SMU Simulated" class="Bool (strict)"("Value"=w221) -> ()  [unwired: 2 in, 2 out]
        n90 = property on="LIA Simulated" class="Bool (strict)"("Value"=w221) -> ()  [unwired: 2 in, 2 out]
        n91 = property on="OPM Simulated" class="Bool (strict)"("Value"=w221) -> ()  [unwired: 2 in, 2 out]
        n92 = call <vilib>:"Add State(s) to Queue__jki_lib_state_machine.vi"("State(s) in (\"\")"=w226) -> ("States Out"=w225:string)  [unwired: 14 in]
      }
      frame "UI: Enable/Disable" {
        n93 = case shown="\"SMU\", Default" w227 {
          frame "SMU", Default {
            n94 = property on="SMU Enable" class="Bool (strict)"() -> ("Value"=w233:bool)  [unwired: 2 in, 2 out]
            n95 = case shown="True" w233 {
              tunnel: [T2."Disabled and Grayed Out" ("Disabled") T2."Enabled" ("Disabled")] -> w232
              frame False {
              }
              frame True {
              }
            }
            n96 = property on="SMU Simulated" class="Bool (strict)"("DisabledEnum"=w232) -> ()  [unwired: 2 in, 2 out]
            n97 = property on="SMU Resource Name" class="VISAName"("DisabledEnum"=w232) -> ()  [unwired: 2 in, 2 out]
            n98 = property on="SMU Channel" class="CmbBox"("DisabledEnum"=w232) -> ()  [unwired: 2 in, 2 out]
          }
          frame "LIA" {
            n99 = property on="LIA Enable" class="Bool (strict)"() -> ("Value"=w237:bool)  [unwired: 2 in, 2 out]
            n100 = case shown="True" w237 {
              tunnel: [T2."Disabled and Grayed Out" ("Disabled") T2."Enabled" ("Disabled")] -> w236
              frame False {
              }
              frame True {
              }
            }
            n101 = property on="LIA Simulated" class="Bool (strict)"("DisabledEnum"=w236) -> ()  [unwired: 2 in, 2 out]
            n102 = property on="LIA Resource Name" class="VISAName"("DisabledEnum"=w236) -> ()  [unwired: 2 in, 2 out]
          }
          frame "OPM" {
            n103 = property on="OPM Enable" class="Bool (strict)"() -> ("Value"=w241:bool)  [unwired: 2 in, 2 out]
            n104 = case shown="True" w241 {
              tunnel: [T2."Disabled and Grayed Out" ("Disabled") T2."Enabled" ("Disabled")] -> w240
              frame False {
              }
              frame True {
              }
            }
            n105 = property on="OPM Simulated" class="Bool (strict)"("DisabledEnum"=w240) -> ()  [unwired: 2 in, 2 out]
            n106 = property on="OPM Resource Name" class="CmbBox"("DisabledEnum"=w240) -> ()  [unwired: 2 in, 2 out]
            n107 = property on="OPM Refresh List" class="Bool (strict)"("DisabledEnum"=w240) -> ()  [unwired: 2 in, 2 out]
          }
          frame "OPA" {
            n108 = property on="OPA Enable" class="Bool (strict)"() -> ("Value"=w245:bool)  [unwired: 2 in, 2 out]
            n109 = case shown="True" w245 {
              tunnel: [T2."Disabled and Grayed Out" ("Disabled") T2."Enabled" ("Disabled")] -> w244
              frame False {
              }
              frame True {
              }
            }
            n110 = property on="OPA Serial Number" class="CmbBox"("DisabledEnum"=w244) -> ()  [unwired: 2 in, 2 out]
            n111 = property on="OPA Refresh List" class="Bool (strict)"("DisabledEnum"=w244) -> ()  [unwired: 2 in, 2 out]
          }
          frame "MC" {
            n112 = property on="MC Enable" class="Bool (strict)"() -> ("Value"=w249:bool)  [unwired: 2 in, 2 out]
            n113 = case shown="True" w249 {
              tunnel: [T2."Disabled and Grayed Out" ("Disabled") T2."Enabled" ("Disabled")] -> w248
              frame False {
              }
              frame True {
              }
            }
            n114 = property on="MC Resource Name" class="VISAName"("DisabledEnum"=w248) -> ()  [unwired: 2 in, 2 out]
          }
          frame "XYStage" {
            n115 = property on="XYStage Enable" class="Bool (strict)"() -> ("Value"=w253:bool)  [unwired: 2 in, 2 out]
            n116 = case shown="True" w253 {
              tunnel: [T2."Disabled and Grayed Out" ("Disabled") T2."Enabled" ("Disabled")] -> w252
              frame False {
              }
              frame True {
              }
            }
            n117 = property on="XYStage Serial Number" class="CmbBox"("DisabledEnum"=w252) -> ()  [unwired: 2 in, 2 out]
            n118 = property on="XYStage Refresh List" class="Bool (strict)"("DisabledEnum"=w252) -> ()  [unwired: 2 in, 2 out]
            n119 = property on="X Axis" class="CmbBox"("DisabledEnum"=w252) -> ()  [unwired: 2 in, 2 out]
            n120 = property on="Y Axis" class="CmbBox"("DisabledEnum"=w252) -> ()  [unwired: 2 in, 2 out]
            n121 = property on="XYStage Enable" class="Bool (strict)"("DisabledEnum"=w252) -> ()  [unwired: 2 in, 2 out]
          }
        }
        n122 = call <vilib>:"Add State(s) to Queue__jki_lib_state_machine.vi"("State(s) in (\"\")"=w231) -> ("States Out"=w230:string)  [unwired: 14 in]
      }
      frame "UI: Tree Init" {
        # "...add new measurement here..."
        # "Select Free mode \nas default"
        n123 = Unbundle By Name(w279) -> ("Measurements Tree"=w278:refnum<vi>)
        n124 = call <instrlib>:"Tree Empty.vi"("Tree Reference In"=w278, "error in (no error)"=w268) -> ("Tree Reference Out"=w280:refnum<vi>, "error out"=w276:errorcluster)  [unwired: 15 in, 1 out]
        n125 = call "Tree Create Measurement Item.vi"("error in (no error)"=w276, "New Text Value"="Free", "TreeControl in"=w280) -> ("error out"=w275:errorcluster, "Created Tag"=w265:string, "TreeControl out"=w277:refnum<vi>)  [unwired: 6 in]
        n126 = call "Tree Create Measurement Item.vi"("error in (no error)"=w275, "New Text Value"=" I/V Curve", "TreeControl in"=w277) -> ("error out"=w272:errorcluster, "TreeControl out"=w273:refnum<vi>)  [unwired: 6 in, 1 out]
        n127 = call "Tree Create Measurement Item.vi"("error in (no error)"=w272, "New Text Value"="Wavelength sweeping", "TreeControl in"=w273) -> ("error out"=w261:errorcluster, "TreeControl out"=w262:refnum<vi>)  [unwired: 6 in, 1 out]
        n128 = call "Tree Create Measurement Item.vi"("error in (no error)"=w261, "New Text Value"="Photocurrent mapping", "TreeControl in"=w262) -> ("error out"=w259:errorcluster, "TreeControl out"=w258:refnum<vi>)  [unwired: 6 in, 1 out]
        n129 = property on="Property Node" class="Tree"(reference=w258, error in=w259) -> (reference out=w271:refnum<vi>, error out=w269:errorcluster, "All Tags"=w270:string[])
        n130 = for {
          tunnel: w270 -> [w287] mode=indexing
          tunnel: w271 -> [w290]
          tunnel: [w286] -> w264
          shift-right: [w283] -> w266
          shift-left: w269 -> [w285]
          n131 = property class="Tree"(reference=w290, error in=w285, "Active Item Tag"=w287) -> (reference out=w289:refnum<vi>, error out=w284:errorcluster, "Child-Only?"=w288:bool)
          n132 = case shown="True" w288 {
            tunnel: w289 -> [w292 w297]
            tunnel: w287 -> [_ w296]
            tunnel: [w292 w295] -> w286
            tunnel: w284 -> [w291 w294]
            tunnel: [w291 w293] -> w283
            frame False {
            }
            frame True {
              n133 = property class="Tree"(reference=w297, error in=w294, "Active Item Tag"=w296, "Glyph"=37, "SelColor"=u32 16777216) -> (reference out=w295:refnum<vi>, error out=w293:errorcluster)
            }
          }
        }
        n134 = property class="Tree"(reference=w264, error in=w266, "Active Item Tag"=w265, "Glyph"=38) -> (error out=w263:errorcluster)  [unwired: 1 out]
        n135 = call <vilib>:"Add State(s) to Queue__jki_lib_state_machine.vi"("State(s) in (\"\")"=w282) -> ("States Out"=w281:string)  [unwired: 14 in]
      }
      frame "UI: Cursor Set" {
        # "Argument"
        # "Set and Unset Cursor Busy.\n(Usage: \"UI: Cursor Set >> Busy|Idle\")"
        n136 = case shown="\"Idle\", Default" w300 {
          tunnel: w302 -> [w307 w309]
          tunnel: [w306 w308] -> w301
          frame "Idle", Default {
            n137 = call <vilib>:"Unset Busy.vi"("error in (no error)"=w307) -> ("error out"=w306:errorcluster)  [unwired: 10 in]
          }
          frame "Busy" {
            n138 = call <vilib>:"Set Busy.vi"("error in (no error)"=w309) -> ("error out"=w308:errorcluster)  [unwired: 9 in, 1 out]
          }
        }
        n139 = call <vilib>:"Add State(s) to Queue__jki_lib_state_machine.vi"("State(s) in (\"\")"=w305) -> ("States Out"=w304:string)  [unwired: 14 in]
      }
      frame "UI: Refresh Devices List" {
        n140 = case shown="\"XYStage\"" w313 {
          tunnel: w312 -> [w318 w323 w328]
          tunnel: [w317 w322 w327] -> w311
          frame "OPA", Default {
            n141 = invoke on="OPA Serial Number" class="CmbBox" method="Reinit To Default"() -> (error out=w319:errorcluster)  [unwired: 3 in, 2 out]
            n142 = call "Locate Devices.vi"("error in (no error)"=w318) -> ("error out"=w317:errorcluster, "Serial Numbers"=w320:string[])  [unwired: 2 in, 1 out]
            n143 = property on="OPA Serial Number" class="CmbBox"(error in=w319, "Strings[]"=w320) -> ()  [unwired: 1 in, 2 out]
            n144 = Index Array(array=w320) -> (element=w321:string)  [unwired: 1 in]
            n145 = property on="OPA Serial Number" class="CmbBox"("Value"=w321) -> ()  [unwired: 2 in, 2 out]
          }
          frame "XYStage" {
            n146 = call "Get MotionControl Devices List.vi"("error in (no error)"=w323) -> ("error out"=w322:errorcluster, "Serial Numbers"=w326:string[])  [unwired: 2 in, 1 out]
            n147 = invoke on="XYStage Serial Number" class="CmbBox" method="Reinit To Default"() -> (error out=w324:errorcluster)  [unwired: 3 in, 2 out]
            n148 = Index Array(array=w326) -> (element=w325:string)  [unwired: 1 in]
            n149 = property on="XYStage Serial Number" class="CmbBox"(error in=w324, "Strings[]"=w326) -> ()  [unwired: 1 in, 2 out]
            n150 = property on="XYStage Serial Number" class="CmbBox"("Value"=w325) -> ()  [unwired: 2 in, 2 out]
          }
          frame "OPM" {
            n151 = invoke on="OPM Resource Name" class="CmbBox" method="Reinit To Default"() -> (error out=w329:errorcluster)  [unwired: 3 in, 2 out]
            n152 = call "Find Resources.vi"("error in (no error)"=w328) -> ("error out"=w327:errorcluster, "Resource Names"=w330:string[])  [unwired: 2 in, 1 out]
            n153 = property on="OPM Resource Name" class="CmbBox"(error in=w329, "Strings[]"=w330) -> ()  [unwired: 1 in, 2 out]
            n154 = Index Array(array=w330) -> (element=w331:string)  [unwired: 1 in]
            n155 = property on="OPM Resource Name" class="CmbBox"("Value"=w331) -> ()  [unwired: 2 in, 2 out]
          }
        }
        n156 = call <vilib>:"Clear Errors.vi"("error in (no error)"=w311) -> ("error out"=w310:errorcluster)  [unwired: 5 in, 1 out]
        n157 = call <vilib>:"Add State(s) to Queue__jki_lib_state_machine.vi"("State(s) in (\"\")"=w316) -> ("States Out"=w315:string)  [unwired: 14 in]
      }
      frame "UI: Front Panel State" {
        # "Argument"
        # "Set Front Panel Open or Closed\n(Usage: \"UI: Front Panel State >> Open|Close\")"
        n158 = Unbundle By Name(w334) -> ("Core.Current VI Reference"=w333:refnum<vi>)
        n159 = case shown="\"Minimize\", \"Minimized\"" w332 {
          tunnel: w336 -> [w344 w359 w370 w383 w396]
          tunnel: [w346 w360 w372 w385 w398] -> w335
          tunnel: w333 -> [w345 w357 w371 w384 w397]
          frame "Open", "Standard", Default {
            w339 = T3."Standard" ("State")
            n160 = property class="VI"(reference=w345, error in=w344) -> (reference out=w342:refnum<vi>, error out=w343:errorcluster, "FP.State"=w341:T3)
            n161 = Not Equal?(x=w341, y=w339) -> (x != y?=w340:bool)
            n162 = case shown="True" w340 {
              tunnel: [w350 w352] -> w346
              tunnel: w343 -> [w349 w352]
              tunnel: w342 -> [w348 _]
              tunnel: w339 -> [w347 _]
              frame True {
                n163 = invoke class="VI" method="FP.Open"(reference=w348, error in=w349, "Activate"=TRUE, "State"=w347) -> (error out=w350:errorcluster)  [unwired: 1 in, 4 out]
              }
              frame False {
              }
            }
          }
          frame "Close", "Closed" {
            n164 = property class="VI"(reference=w357, error in=w359) -> (reference out=w356:refnum<vi>, error out=w358:errorcluster, "FP.State"=w354:T3)
            n165 = Not Equal?(x=w354, y=T3."Closed" ("Front Panel Window:State")) -> (x != y?=w353:bool)
            n166 = case shown="True" w353 {
              tunnel: [w361 w364] -> w360
              tunnel: w358 -> [w361 w363]
              tunnel: w356 -> [_ w362]
              frame False {
              }
              frame True {
                n167 = invoke class="VI" method="FP.Close"(reference=w362, error in=w363) -> (error out=w364:errorcluster)  [unwired: 1 in, 2 out]
              }
            }
          }
          frame "Hidden", "Hide" {
            w365 = T3."Hidden" ("State")
            n168 = property class="VI"(reference=w371, error in=w370) -> (reference out=w368:refnum<vi>, error out=w369:errorcluster, "FP.State"=w367:T3)
            n169 = Not Equal?(x=w367, y=w365) -> (x != y?=w366:bool)
            n170 = case shown="True" w366 {
              tunnel: [w376 w377] -> w372
              tunnel: w369 -> [w375 w377]
              tunnel: w368 -> [w374 _]
              tunnel: w365 -> [w373 _]
              frame True {
                n171 = invoke class="VI" method="FP.Open"(reference=w374, error in=w375, "State"=w373) -> (error out=w376:errorcluster)  [unwired: 2 in, 4 out]
              }
              frame False {
              }
            }
          }
          frame "Minimize", "Minimized" {
            w378 = T3."Minimized" ("State")
            n172 = property class="VI"(reference=w384, error in=w383) -> (reference out=w381:refnum<vi>, error out=w382:errorcluster, "FP.State"=w380:T3)
            n173 = Not Equal?(x=w380, y=w378) -> (x != y?=w379:bool)
            n174 = case shown="True" w379 {
              tunnel: [w389 w390] -> w385
              tunnel: w382 -> [w388 w390]
              tunnel: w381 -> [w387 _]
              tunnel: w378 -> [w386 _]
              frame True {
                n175 = invoke class="VI" method="FP.Open"(reference=w387, error in=w388, "State"=w386) -> (error out=w389:errorcluster)  [unwired: 2 in, 4 out]
              }
              frame False {
              }
            }
          }
          frame "Maximize", "Maximized" {
            w391 = T3."Maximized" ("State")
            n176 = property class="VI"(reference=w397, error in=w396) -> (reference out=w394:refnum<vi>, error out=w395:errorcluster, "FP.State"=w393:T3)
            n177 = Not Equal?(x=w393, y=w391) -> (x != y?=w392:bool)
            n178 = case shown="True" w392 {
              tunnel: [w402 w403] -> w398
              tunnel: w395 -> [w401 w403]
              tunnel: w394 -> [w400 _]
              tunnel: w391 -> [w399 _]
              frame True {
                n179 = invoke class="VI" method="FP.Open"(reference=w400, error in=w401, "State"=w399) -> (error out=w402:errorcluster)  [unwired: 2 in, 4 out]
              }
              frame False {
              }
            }
          }
        }
        n180 = call <vilib>:"Add State(s) to Queue__jki_lib_state_machine.vi"("State(s) in (\"\")"=w338) -> ("States Out"=w337:string)  [unwired: 14 in]
      }
      frame "UI: Select Type" {
        n181 = case shown="\"Photocurrent mapping\"" w432 {
          tunnel: w431 -> [w444 w455 w464 w477]
          tunnel: [w442 w454 w465 w476] -> w430
          tunnel: [w434 w450 w461 w472] -> w425
          tunnel: [w439 w449 w460 w471] -> w421
          tunnel: [w438 w448 w459 w470] -> w417
          tunnel: [w437 w447 w458 w469] -> w413
          tunnel: [w436 w446 w457 w468] -> w409
          tunnel: [w435 w445 w456 w467] -> w405
          frame "Free", Default {
            w435 = T2."Enabled"  # MC
            w436 = T2."Enabled"  # XYStage
            w437 = T2."Enabled"  # OPA
            w438 = T2."Enabled"  # OPM
            w439 = T2."Enabled"  # LIA
            w434 = T2."Enabled"  # SMU
            n182 = Bundle By Name(cluster=w444, "Measurement.Type"=Measurement.Type--Enum."Free") -> (w442:T23)
            n183 = property on="Measurement Parameters" class="TabCtl (strict)"("Value"=T1."Free" ("Measurement Parameters")) -> ()  [unwired: 2 in, 2 out]
            n184 = property on="Status" class="Str"("Value"="Free measurement mode" ("Status")) -> ()  [unwired: 2 in, 2 out]
          }
          frame "I/V Curve" {
            w445 = T2."Disabled and Grayed Out"  # MC
            w446 = T2."Disabled and Grayed Out"  # XYStage
            w447 = T2."Disabled and Grayed Out"  # OPA
            w448 = T2."Disabled and Grayed Out"  # OPM
            w449 = T2."Disabled and Grayed Out"  # LIA
            w450 = T2."Enabled"  # SMU
            n185 = Bundle By Name(cluster=w455, "Measurement.Type"=Measurement.Type--Enum."I/V Curve") -> (w454:T23)
            n186 = property on="Measurement Parameters" class="TabCtl (strict)"("Value"=T1."I-V Curve" ("Measurement Parameters")) -> ()  [unwired: 2 in, 2 out]
            n187 = property on="Status" class="Str"("Value"="I/V curve measurement mode" ("Status")) -> ()  [unwired: 2 in, 2 out]
          }
          frame "Wavelength sweeping" {
            w456 = T2."Enabled"  # MC
            w457 = T2."Disabled and Grayed Out"  # XYStage
            w458 = T2."Enabled"  # OPA
            w459 = T2."Enabled"  # OPM
            w460 = T2."Enabled"  # LIA
            w461 = T2."Enabled"  # SMU
            n188 = Bundle By Name(cluster=w464, "Measurement.Type"=Measurement.Type--Enum."Wavelength sweeping") -> (w465:T23)
            n189 = property on="Measurement Parameters" class="TabCtl (strict)"("Value"=T1."Wavelength Sweeping" ("Measurement Parameters")) -> ()  [unwired: 2 in, 2 out]
            n190 = property on="Status" class="Str"("Value"=" Wavelength Sweeping measurement mode" ("Status")) -> ()  [unwired: 2 in, 2 out]
          }
          frame "Photocurrent mapping" {
            w467 = T2."Disabled and Grayed Out"  # MC
            w468 = T2."Enabled"  # XYStage
            w469 = T2."Disabled and Grayed Out"  # OPA
            w470 = T2."Disabled and Grayed Out"  # OPM
            w471 = T2."Enabled"  # LIA
            w472 = T2."Enabled"  # SMU
            n191 = Bundle By Name(cluster=w477, "Measurement.Type"=Measurement.Type--Enum."Photocurrent mapping") -> (w476:T23)
            n192 = property on="Measurement Parameters" class="TabCtl (strict)"("Value"=T1."Photocurrent mapping" ("Measurement Parameters")) -> ()  [unwired: 2 in, 2 out]
            n193 = property on="Status" class="Str"("Value"=" Photocurrent mapping measurement mode" ("Status")) -> ()  [unwired: 2 in, 2 out]
          }
        }
        n194 = property on="OPA Enable" class="Bool (strict)"() -> ("Value"=w414:bool)  [unwired: 2 in, 2 out]
        n195 = property on="XYStage Enable" class="Bool (strict)"() -> ("Value"=w411:bool)  [unwired: 2 in, 2 out]
        n196 = property on="LIA Enable" class="Bool (strict)"() -> ("Value"=w422:bool)  [unwired: 2 in, 2 out]
        n197 = property on="OPM Enable" class="Bool (strict)"() -> ("Value"=w418:bool)  [unwired: 2 in, 2 out]
        n198 = property on="SMU Enable" class="Bool (strict)"() -> ("Value"=w427:bool)  [unwired: 2 in, 2 out]
        n199 = property on="MC Enable" class="Bool (strict)"() -> ("Value"=w407:bool)  [unwired: 2 in, 2 out]
        n200 = call "Bool To Disabled.vi"("Bool"=w411) -> ("Disabled"=w410:T2)
        n201 = call "Bool To Disabled.vi"("Bool"=w414) -> ("Disabled"=w415:T2)
        n202 = call "Bool To Disabled.vi"("Bool"=w422) -> ("Disabled"=w423:T2)
        n203 = call "Bool To Disabled.vi"("Bool"=w418) -> ("Disabled"=w419:T2)
        n204 = call "Bool To Disabled.vi"("Bool"=w427) -> ("Disabled"=w426:T2)
        n205 = call "Bool To Disabled.vi"("Bool"=w407) -> ("Disabled"=w406:T2)
        n206 = call "Disabled And.vi"("Disabled 2"=w410, "Disabled 1"=w409) -> ("Disabled"=w408:T2)
        n207 = call "Disabled And.vi"("Disabled 2"=w415, "Disabled 1"=w413) -> ("Disabled"=w412:T2)
        n208 = call "Disabled And.vi"("Disabled 2"=w423, "Disabled 1"=w421) -> ("Disabled"=w420:T2)
        n209 = call "Disabled And.vi"("Disabled 2"=w419, "Disabled 1"=w417) -> ("Disabled"=w416:T2)
        n210 = call "Disabled And.vi"("Disabled 2"=w426, "Disabled 1"=w425) -> ("Disabled"=w424:T2)
        n211 = call "Disabled And.vi"("Disabled 2"=w406, "Disabled 1"=w405) -> ("Disabled"=w404:T2)
        n212 = property on="SMU Simulated" class="Bool (strict)"("DisabledEnum"=w424) -> ()  [unwired: 2 in, 2 out]
        n213 = property on="SMU Resource Name" class="VISAName"("DisabledEnum"=w424) -> ()  [unwired: 2 in, 2 out]
        n214 = property on="SMU Channel" class="CmbBox"("DisabledEnum"=w424) -> ()  [unwired: 2 in, 2 out]
        n215 = property on="LIA Simulated" class="Bool (strict)"("DisabledEnum"=w420) -> ()  [unwired: 2 in, 2 out]
        n216 = property on="LIA Resource Name" class="VISAName"("DisabledEnum"=w420) -> ()  [unwired: 2 in, 2 out]
        n217 = property on="OPM Simulated" class="Bool (strict)"("DisabledEnum"=w416) -> ()  [unwired: 2 in, 2 out]
        n218 = property on="OPM Resource Name" class="CmbBox"("DisabledEnum"=w416) -> ()  [unwired: 2 in, 2 out]
        n219 = property on="OPM Refresh List" class="Bool (strict)"("DisabledEnum"=w416) -> ()  [unwired: 2 in, 2 out]
        n220 = property on="OPA Serial Number" class="CmbBox"("DisabledEnum"=w412) -> ()  [unwired: 2 in, 2 out]
        n221 = property on="OPA Refresh List" class="Bool (strict)"("DisabledEnum"=w412) -> ()  [unwired: 2 in, 2 out]
        n222 = property on="XYStage Serial Number" class="CmbBox"("DisabledEnum"=w408) -> ()  [unwired: 2 in, 2 out]
        n223 = property on="XYStage Refresh List" class="Bool (strict)"("DisabledEnum"=w408) -> ()  [unwired: 2 in, 2 out]
        n224 = property on="X Axis" class="CmbBox"("DisabledEnum"=w408) -> ()  [unwired: 2 in, 2 out]
        n225 = property on="Y Axis" class="CmbBox"("DisabledEnum"=w408) -> ()  [unwired: 2 in, 2 out]
        n226 = property on="MC Resource Name" class="VISAName"("DisabledEnum"=w404) -> ()  [unwired: 2 in, 2 out]
        n227 = property on="SMU Enable" class="Bool (strict)"("DisabledEnum"=w425) -> ()  [unwired: 2 in, 2 out]
        n228 = property on="LIA Enable" class="Bool (strict)"("DisabledEnum"=w421) -> ()  [unwired: 2 in, 2 out]
        n229 = property on="OPM Enable" class="Bool (strict)"("DisabledEnum"=w417) -> ()  [unwired: 2 in, 2 out]
        n230 = property on="OPA Enable" class="Bool (strict)"("DisabledEnum"=w413) -> ()  [unwired: 2 in, 2 out]
        n231 = property on="XYStage Enable" class="Bool (strict)"("DisabledEnum"=w409) -> ()  [unwired: 2 in, 2 out]
        n232 = property on="MC Enable" class="Bool (strict)"("DisabledEnum"=w405) -> ()  [unwired: 2 in, 2 out]
        n233 = call <vilib>:"Add State(s) to Queue__jki_lib_state_machine.vi"("State(s) in (\"\")"=w429) -> ("States Out"=w433:string)  [unwired: 14 in]
      }
      frame "---------- Macro ----------" {
        # "Do not put any code in this frame.\n(It is a separator no-op. You can make a copy of this frame to create a new Macro frame)"
        n234 = call <vilib>:"Add State(s) to Queue__jki_lib_state_machine.vi"("State(s) in (\"\")"=w481) -> ("States Out"=w480:string)  [unwired: 14 in]
      }
      frame "Macro: Initialize" {
        # "Initialization Macro\n(This is called once, when the VI starts)"
        n235 = call <vilib>:"Add State(s) to Queue__jki_lib_state_machine.vi"("State(s) in Front (\"\")"="Data: Initialize\nInitialize Core Data\nUI: Initialize\nUI: Front Panel State >> Open", "State(s) in (\"\")"=w486) -> ("States Out"=w485:string)  [unwired: 13 in]
      }
      frame "Macro: Exit" {
        # "Exit Macro\n(This is called once, when the VI exits)"
        n236 = Unbundle By Name(w493) -> ("Core.Close Panel on Exit?"=w492:bool)
        n237 = Select(t="UI: Front Panel State >> Close", s=w492, f="") -> (s? t:f=w489:string)
        n238 = call <vilib>:"Add State(s) to Queue__jki_lib_state_machine.vi"("State(s) in (\"\")"=w489, "State(s) at Back (\"\")"="Data: Cleanup\nExit") -> ("States Out"=w487:string)  [unwired: 13 in]
        n239 = call <vilib>:"Add State(s) to Queue__jki_lib_state_machine.vi"("State(s) in Front (\"\")"=w487, "State(s) in (\"\")"=w496) -> ("States Out"=w495:string)  [unwired: 13 in]
      }
      frame "---------- Measurements ----------" {
        # "Template Separator\n(You can make a copy of, or modify, this frame)"
        n240 = call <vilib>:"Add State(s) to Queue__jki_lib_state_machine.vi"("State(s) in (\"\")"=w500) -> ("States Out"=w499:string)  [unwired: 14 in]
      }
      frame "Measurements: Start" {
        n241 = Unbundle By Name(w507) -> ("Measurement.Type"=w506:T5, "Configuration (variant)"=w501:variant)
        n242 = case shown="\"Free\", Default" w506 {
          tunnel: [w511 w512 w515 w516] -> w505
          tunnel: [w510 w513 w514 w517] -> w504
          frame "Free", Default {
            w510 = refnum<class "Measurement.Free.UI.lvclass"> refnum  # Measurement.Free.UI
            w511 = refnum<class "Measurement.Free.lvclass"> refnum  # Measurement.Free
          }
          frame "I/V Curve" {
            w513 = refnum<class "Measurement.IVCurve.UI.lvclass"> refnum  # Measurement.IVCurve.UI
            w512 = refnum<class "Measurement.IVCurve.lvclass"> refnum  # Measurement.IVCurve
          }
          frame "Wavelength sweeping" {
            w514 = refnum<class "Measurement.WavelengthSweeping.UI.lvclass"> refnum  # Measurement.WavelengthSweeping.UI
            w515 = refnum<class "Measurement.WavelengthSweeping.lvclass"> refnum  # Measurement.WavelengthSweeping
          }
          frame "Photocurrent mapping" {
            w517 = refnum<class "Measurement.PhotocurrentMapping.UI.lvclass"> refnum  # Measurement.PhotocurrentMapping.UI
            w516 = refnum<class "Measurement.PhotocurrentMapping.lvclass"> refnum  # Measurement.PhotocurrentMapping
          }
        }
        n243 = call "Measurement Launcher.vi"("error in (no error)"=w503, "Configuration"=w501, "Measurement.UI"=w504, "Measurement"=w505) -> ("error out"=w502:errorcluster)  [unwired: 7 in]
        n244 = call <vilib>:"Add State(s) to Queue__jki_lib_state_machine.vi"("State(s) in (\"\")"=w509) -> ("States Out"=w508:string)  [unwired: 14 in]
      }
      frame "---------- Configuration ----------" {
        # "Do not put any code in this frame.\n(it is a separator no-op)"
        n245 = call <vilib>:"Add State(s) to Queue__jki_lib_state_machine.vi"("State(s) in (\"\")"=w521) -> ("States Out"=w520:string)  [unwired: 14 in]
      }
      frame "Configuration: Create" {
        n246 = Unbundle By Name(w524) -> ("Measurement.Type"=w523:T5)
        n247 = case shown="\"Free\", Default" w523 {
          tunnel: ["Configuration: Create Part >> SMU\nConfiguration: Create Part >> LIA\nConfiguration: Create Part >> OPM\nConfiguration: Create Part >> OPA\nConfiguration: Create Part >> MC\nConfiguration: Create Part >> Free\nConfiguration: Create Main >> Free" ("State(s) in Front (\"\")") "Configuration: Create Part >> SMU\nConfiguration: Create Part >> I/V Curve\nConfiguration: Create Main >> I/V Curve" ("State(s) in Front (\"\")") "Configuration: Create Part >> SMU\nConfiguration: Create Part >> LIA\nConfiguration: Create Part >> OPM\nConfiguration: Create Part >> OPA\nConfiguration: Create Part >> MC\nConfiguration: Create Part >> Wavelength sweeping\nConfiguration: Create Main >> Wavelength sweeping" ("State(s) in Front (\"\")") "Configuration: Create Part >> SMU\nConfiguration: Create Part >> LIA\nConfiguration: Create Part >> XYStage\nConfiguration: Create Part >> Photocurrent mapping\nConfiguration: Create Main >> Photocurrent mapping" ("State(s) in Front (\"\")")] -> w522
          frame "Free", Default {
          }
          frame "I/V Curve" {
          }
          frame "Wavelength sweeping" {
          }
          frame "Photocurrent mapping" {
          }
        }
        n248 = call <vilib>:"Add State(s) to Queue__jki_lib_state_machine.vi"("State(s) in Front (\"\")"=w522, "State(s) in (\"\")"=w527) -> ("States Out"=w526:string)  [unwired: 13 in]
      }
      frame "Configuration: Create Part" {
        n249 = case shown="\"XYStage\"" w534 {
          tunnel: w533 -> [w540 w552 w564 w568 w579 w593 w594 w596 w607 w631]
          tunnel: [w539 w551 w563 w569 w578 w592 w594 w597 w606 w630] -> w532
          frame "SMU", Default {
            w544 = T7 {"Enable"=FALSE, "SMU Model"="", "Configuration"={"VISA Resource"="", "Channel"=""}}  # Configuration.SMU
            n250 = property on="SMU Simulated" class="Bool (strict)"() -> ("Value"=w542:bool)  [unwired: 2 in, 2 out]
            n251 = case shown="True" w542 {
              tunnel: ["Keithley2600" ("SMU Model") "Simulated" ("SMU Model")] -> w543
              frame False {
              }
              frame True {
              }
            }
            n252 = property on="SMU Resource Name" class="VISAName"() -> ("Value"=w545:refnum<visa-resource-name>)  [unwired: 2 in, 2 out]
            n253 = property on="SMU Channel" class="CmbBox"() -> ("Value"=w546:string)  [unwired: 2 in, 2 out]
            n254 = Bundle By Name(cluster=w544, "Enable"="SMU Enable", "SMU Model"=w543, "Configuration.VISA Resource"=w545, "Configuration.Channel"=w546) -> (w541:T7)
            n255 = Bundle By Name(cluster=w540, "Configuration.Hardware.SMU"=w541) -> (w539:T23)
          }
          frame "LIA" {
            w553 = T9 {"Enable"=FALSE, "LIA Model"="", "Configuration"={"VISA Resource"=""}}  # Configuration.LIA
            n256 = property on="LIA Simulated" class="Bool (strict)"() -> ("Value"=w556:bool)  [unwired: 2 in, 2 out]
            n257 = case shown="False" w556 {
              tunnel: ["SR810" ("SMU Model") "Simulated" ("SMU Model")] -> w554
              frame False {
              }
              frame True {
              }
            }
            n258 = property on="LIA Resource Name" class="VISAName"() -> ("Value"=w555:refnum<visa-resource-name>)  [unwired: 2 in, 2 out]
            n259 = Bundle By Name(cluster=w553, "Enable"="LIA Enable", "LIA Model"=w554, "Configuration.VISA Resource"=w555) -> (w550:T9)
            n260 = Bundle By Name(cluster=w552, "Configuration.Hardware.LIA"=w550) -> (w551:T23)
          }
          frame "MC" {
            w561 = T17 {"Enable"=FALSE, "MC Model"="", "Configuration"={"VISA Resource"=""}}  # Configuration.MC
            n261 = property on="MC Resource Name" class="VISAName"() -> ("Value"=w560:refnum<visa-resource-name>)  [unwired: 2 in, 2 out]
            n262 = Bundle By Name(cluster=w561, "Enable"="MC Enable", "MC Model"="DangwooOptron" ("SMU Model"), "Configuration.VISA Resource"=w560) -> (w562:T17)
            n263 = Bundle By Name(cluster=w564, "Configuration.Hardware.MC"=w562) -> (w563:T23)
          }
          frame "OPM" {
            w570 = T11 {"Enable"=FALSE, "OPM Model"="", "Configuration"={"VISA Resource"=""}}  # Configuration.OPM
            n264 = property on="OPM Simulated" class="Bool (strict)"() -> ("Value"=w573:bool)  [unwired: 2 in, 2 out]
            n265 = case shown="False" w573 {
              tunnel: ["ThorlabsPM400" ("SMU Model") "Simulated" ("SMU Model")] -> w571
              frame False {
              }
              frame True {
              }
            }
            n266 = property on="OPM Resource Name" class="CmbBox"() -> ("Value"=w572:string)  [unwired: 2 in, 2 out]
            n267 = Bundle By Name(cluster=w570, "Enable"="OPM Enable", "OPM Model"=w571, "Configuration.VISA Resource"=w572) -> (w567:T11)
            n268 = Bundle By Name(cluster=w568, "Configuration.Hardware.OPM"=w567) -> (w569:T23)
          }
          frame "OPA" {
            w581 = T13 {"Enable"=FALSE, "OPA Model"="", "Configuration"={"Serial Number"=""}}  # Configuration.OPA
            n269 = property on="OPA Serial Number" class="CmbBox"() -> ("Value"=w582:string)  [unwired: 2 in, 2 out]
            n270 = Bundle By Name(cluster=w581, "Enable"="OPA Enable", "OPA Model"="OrpheusHP", "Configuration.Serial Number"=w582) -> (w577:T13)
            n271 = Bundle By Name(cluster=w579, "Configuration.Hardware.OPA"=w577) -> (w578:T23)
          }
          frame "XYStage" {
            w591 = T15 {"Enable"=FALSE, "XYStage Model"="", "Configuration"={"Serial Number"="", "X Axis"="", "Y Axis"="", "Real-World Units"="", "Counts per Unit"=1}}  # Configuration.XYStage
            n272 = property on="XYStage Serial Number" class="CmbBox"() -> ("Value"=w588:string)  [unwired: 2 in, 2 out]
            n273 = Bundle By Name(cluster=w591, "Enable"="XYStage Enable", "XYStage Model"="KIM101", "Configuration.Serial Number"=w588, "Configuration.X Axis"="X Axis", "Configuration.Y Axis"="Y Axis", "Configuration.Real-World Units"="Real world units", "Configuration.Counts per Unit"="Counts per unit") -> (w590:T15)
            n274 = Bundle By Name(cluster=w593, "Configuration.Hardware.XYStage"=w590) -> (w592:T23)
          }
          frame "Free" {
            # "Create Free measurement configuration"
            # "Nothing to do"
          }
          frame "I/V Curve" {
            w603 = T19 {"SMU Voltage Start, V"=0.0, "SMU Voltage Stop, V"=0.0, "SMU Voltage Step, V"=0.0, "Delay time, ms"=0, "Accumulation"=0}  # Configuration.Measurement
            # "Create I/V Curve measurement configuration"
            n275 = Bundle By Name(cluster=w603, "SMU Voltage Start, V"="SMU start voltage, V", "SMU Voltage Stop, V"="SMU stop voltage, V", "SMU Voltage Step, V"="SMU step voltage, V", "Delay time, ms"="Delay time, ms", "Accumulation"="I/V Curve Accumulation") -> (w595:T19)
            n276 = Bundle By Name(cluster=w596, "Configuration.Measurement.I/V Curve"=w595) -> (w597:T23)
          }
          frame "Wavelength sweeping" {
            w608 = T20 {"SMU Voltage, V"=0.0, "Start wavelength, nm"=0.0, "Stop wavelength, nm"=0.0, "Scan resolution, nm"=0.0, "Number or points"=0, "Integration time, sec"=0.0, "Delay time, ms"=0, "Accumulation"=0, "Wavelength offset, nm"=0.0}  # Configuration.Measurement
            # "Create Wavelength sweeping measurement configuration"
            n277 = Bundle By Name(cluster=w608, "SMU Voltage, V"="SMU voltage, V", "Start wavelength, nm"="Start wavelength, nm", "Stop wavelength, nm"="Stop wavelength, nm", "Scan resolution, nm"="Scan resolution, nm", "Number or points"="OPA number of points", "Integration time, sec"="Integration time, s", "Delay time, ms"="Delay time, ms", "Accumulation"="W-Sweep Accumulation", "Wavelength offset, nm"="Monochromator\nwavelength offset, nm") -> (w605:T20)
            n278 = Bundle By Name(cluster=w607, "Configuration.Measurement.W-Sweep"=w605) -> (w606:T23)
          }
          frame "Photocurrent mapping" {
            w617 = T21 {"X"={"Start, units"=-10000.0, "Stop, units"=10000.0, "Step, units"=250.0}, "Y"={"Start, units"=-10000.0, "Stop, units"=10000.0, "Step, units"=250.0}, "Accumulation"=5}  # Configuration.Measurement
            w628 = T22 {"Start, units"=-10000.0, "Stop, units"=10000.0, "Step, units"=250.0}  # Configuration.Axis
            w629 = T22 {"Start, units"=-10000.0, "Stop, units"=10000.0, "Step, units"=250.0}  # Configuration.Axis
            # "Create Photocurrent mapping measurement configuration"
            n279 = Bundle By Name(cluster=w629, "Start, units"="X Axis Start, units", "Stop, units"="X Axis Stop, units", "Step, units"="X Axis Step, units") -> (w620:T22)
            n280 = Bundle By Name(cluster=w628, "Start, units"="Y Axis Start, units", "Stop, units"="Y Axis Stop, units", "Step, units"="Y Axis Step, units") -> (w619:T22)
            n281 = Bundle By Name(cluster=w617, "X"=w620, "Y"=w619, "Accumulation"="P-Map Accumulation") -> (w621:T21)
            n282 = Bundle By Name(cluster=w631, "Configuration.Measurement.P-Map"=w621) -> (w630:T23)
          }
        }
        n283 = call <vilib>:"Add State(s) to Queue__jki_lib_state_machine.vi"("State(s) in (\"\")"=w537) -> ("States Out"=w536:string)  [unwired: 14 in]
      }
      frame "Configuration: Create Main" {
        n284 = case shown="\"Free\", Default" w634 {
          tunnel: w633 -> [w642 w653 w662 w673]
          tunnel: [w641 w654 w661 w674] -> w632
          frame "Free", Default {
            w648 = T26 {"Measurement.Type"=enum."Free", "Hardware"={"SMU"={"Enable"=FALSE, "SMU Model"="", "Configuration"={"VISA Resource"="", "Channel"=""}}, "LIA"={"Enable"=FALSE, "LIA Model"="", "Configuration"={"VISA Resource"=""}}, "OPM"={"Enable"=FALSE, "OPM Model"="", "Configuration"={"VISA Resource"=""}}, "OPA"={"Enable"=FALSE, "OPA Model"="", "Configuration"={"Serial Number"=""}}, "MC"={"Enable"=FALSE, "MC Model"="", "Configuration"={"VISA Resource"=""}}}}  # Configuration
            n285 = Unbundle By Name(w642) -> ("Configuration.Hardware.SMU"=w646:T7, "Configuration.Hardware.LIA"=w645:T9, "Configuration.Hardware.OPM"=w644:T11, "Configuration.Hardware.OPA"=w643:T13, "Configuration.Hardware.MC"=w638:T17)
            n286 = Bundle By Name(cluster=w648, "Measurement.Type"=Measurement.Type--Enum."Free", "Hardware.SMU"=w646, "Hardware.LIA"=w645, "Hardware.OPM"=w644, "Hardware.OPA"=w643, "Hardware.MC"=w638) -> (w640:T26)
            n287 = To Variant(anything=w640) -> (Variant=w639:variant)
            n288 = Bundle By Name(cluster=w642, "Configuration (variant)"=w639) -> (w641:T23)
          }
          frame "I/V Curve" {
            w652 = T28 {"Measurement.Type"=enum."Free", "Hardware"={"SMU"={"Enable"=FALSE, "SMU Model"="", "Configuration"={"VISA Resource"="", "Channel"=""}}}, "Measurement"={"SMU Voltage Start, V"=0.0, "SMU Voltage Stop, V"=0.0, "SMU Voltage Step, V"=0.0, "Delay time, ms"=0, "Accumulation"=0}}  # Configuration
            n289 = Unbundle By Name(w653) -> ("Configuration.Hardware.SMU"=w655:T7, "Configuration.Measurement.I/V Curve"=w651:T19)
            n290 = Bundle By Name(cluster=w652, "Measurement.Type"=Measurement.Type--Enum."I/V Curve", "Hardware.SMU"=w655, "Measurement"=w651) -> (w650:T28)
            n291 = To Variant(anything=w650) -> (Variant=w649:variant)
            n292 = Bundle By Name(cluster=w653, "Configuration (variant)"=w649) -> (w654:T23)
          }
          frame "Wavelength sweeping" {
            w668 = T30 {"Measurement.Type"=enum."Free", "Hardware"={"SMU"={"Enable"=FALSE, "SMU Model"="", "Configuration"={"VISA Resource"="", "Channel"=""}}, "LIA"={"Enable"=FALSE, "LIA Model"="", "Configuration"={"VISA Resource"=""}}, "OPM"={"Enable"=FALSE, "OPM Model"="", "Configuration"={"VISA Resource"=""}}, "OPA"={"Enable"=FALSE, "OPA Model"="", "Configuration"={"Serial Number"=""}}, "MC"={"Enable"=FALSE, "MC Model"="", "Configuration"={"VISA Resource"=""}}}, "Measurement"={"SMU Voltage, V"=0.0, "Start wavelength, nm"=0.0, "Stop wavelength, nm"=0.0, "Scan resolution, nm"=0.0, "Number or points"=0, "Integration time, sec"=0.0, "Delay time, ms"=0, "Accumulation"=0, "Wavelength offset, nm"=0.0}}  # Configuration
            n293 = Unbundle By Name(w662) -> ("Configuration.Hardware.SMU"=w667:T7, "Configuration.Hardware.LIA"=w666:T9, "Configuration.Hardware.OPM"=w665:T11, "Configuration.Hardware.OPA"=w664:T13, "Configuration.Hardware.MC"=w657:T17, "Configuration.Measurement.W-Sweep"=w663:T20)
            n294 = Bundle By Name(cluster=w668, "Measurement.Type"=Measurement.Type--Enum."Wavelength sweeping", "Hardware.SMU"=w667, "Hardware.LIA"=w666, "Hardware.OPM"=w665, "Hardware.OPA"=w664, "Hardware.MC"=w657, "Measurement"=w663) -> (w659:T30)
            n295 = To Variant(anything=w659) -> (Variant=w658:variant)
            n296 = Bundle By Name(cluster=w662, "Configuration (variant)"=w658) -> (w661:T23)
          }
          frame "Photocurrent mapping" {
            w670 = T32 {"Measurement.Type"=enum."Free", "Hardware"={"SMU"={"Enable"=FALSE, "SMU Model"="", "Configuration"={"VISA Resource"="", "Channel"=""}}, "LIA"={"Enable"=FALSE, "LIA Model"="", "Configuration"={"VISA Resource"=""}}, "XYStage"={"Enable"=FALSE, "XYStage Model"="", "Configuration"={"Serial Number"="", "X Axis"="", "Y Axis"="", "Real-World Units"="", "Counts per Unit"=1}}}, "Measurement"={"X"={"Start, units"=-10000.0, "Stop, units"=10000.0, "Step, units"=250.0}, "Y"={"Start, units"=-10000.0, "Stop, units"=10000.0, "Step, units"=250.0}, "Accumulation"=5}}  # Configuration
            n297 = Unbundle By Name(w673) -> ("Configuration.Hardware.SMU"=w677:T7, "Configuration.Hardware.LIA"=w676:T9, "Configuration.Hardware.XYStage"=w669:T15, "Configuration.Measurement.P-Map"=w675:T21)
            n298 = Bundle By Name(cluster=w670, "Measurement.Type"=Measurement.Type--Enum."Photocurrent mapping", "Hardware.SMU"=w677, "Hardware.LIA"=w676, "Hardware.XYStage"=w669, "Measurement"=w675) -> (w672:T32)
            n299 = To Variant(anything=w672) -> (Variant=w671:variant)
            n300 = Bundle By Name(cluster=w673, "Configuration (variant)"=w671) -> (w674:T23)
          }
        }
        n301 = call <vilib>:"Add State(s) to Queue__jki_lib_state_machine.vi"("State(s) in (\"\")"=w637) -> ("States Out"=w636:string)  [unwired: 14 in]
      }
    }
  }
